vi "NIMS_NS_fir_nyquist.vi"(5 "Function name":string, 6 "Line number":i32, 7 "Number of outputs requested":i32, 8 "error in (no error)":errorcluster, 11 "[A]":variant[](array[variant])) -> (0 "error out":errorcluster, 3 "[funct(A)]":variant[](array[variant]))   [LabVIEW 2017]
uses:
  <vilib>/imath/engines/lvmath/Functions/Error Handling/error.ctl
  <instcachedir>/0/NIMS_RunTimeType_From StrictType (excl LVString)_1019F277F0A747EDBCA0F6C52CA54500.lvgen/NIMS_RunTimeType_From StrictType (excl LVString)_1019F277F0A747EDBCA0F6C52CA54500_000.vi
  <instcachedir>/0/NIMS_Get Row Vector_w Error - Matrix_7ECCFA0649AF47C08F6F0C496599EB01.lvgen/NIMS_Get Row Vector_w Error - Matrix_7ECCFA0649AF47C08F6F0C496599EB01_000.vi
  <instcachedir>/0/NIMS_Get Scalar_w Error_1987D997E87247DDAC16EA23A5E9E4FC.lvgen/NIMS_Get Scalar_w Error_1987D997E87247DDAC16EA23A5E9E4FC_000.vi
  <instcachedir>/0/NIMS_Get Scalar_w Error_1987D997E87247DDAC16EA23A5E9E4FC.lvgen/NIMS_Get Scalar_w Error_1987D997E87247DDAC16EA23A5E9E4FC_003.vi
  <instcachedir>/0/NIMS_Complex To Real_BE01396FDE034E8E94CEBBA1E368668D.lvgen/NIMS_Complex To Real_BE01396FDE034E8E94CEBBA1E368668D_000.vi
  <instcachedir>/0/NIMS_Get Row Vector_w Error - Matrix_7ECCFA0649AF47C08F6F0C496599EB01.lvgen/NIMS_Get Row Vector_w Error - Matrix_7ECCFA0649AF47C08F6F0C496599EB01_001.vi
  <instcachedir>/0/NIMS_RunTimeType_To Numeric_1CBDAFC4EFAD4045A1DE52278D16738D.lvgen/NIMS_RunTimeType_To Numeric_1CBDAFC4EFAD4045A1DE52278D16738D_000.vi
  <vilib>/addons/Digital Filter Design/NI_DigFilter_MathScript.lvlib
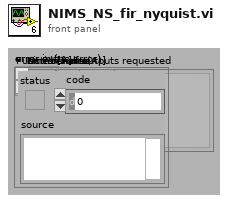
[diagram p1: front panel]
types:
  T1 = typedef "error.ctl" = enum16{"No Error", "Problem", "Input type must not be void", "Incorrect number of parameters", "Function not defined for non-numeric types", "An output variable of the user-defined function is undefined", "Function only defined for character arrays", "Function not defined for boolean, character, or single precision", "Function not defined for complex types", "Not a valid operation", "Inputs must be scalar", "Input matrices are not the same size", "Function only available on RT", "Input matrices must be nonnegative integers of the same type", "Arguments must be non-negative integers less than bitmax", "Number to complement must be less than 2^N", "Bit to get is outside range", "Bit to set is outside range", "Input must be real type ", "At least one parameter must be scalar", "Unable to display plug-in data on RT", "Function not defined for higher dimensional matrices", "Invalid attributes", "Wrong Type of Input Arguments", "Wrong Argument Option", "Invalid file identifier", "Indices must be real positive integers", "The variable is not a matrix data type.", "Number of elements must be the same for indices and values", "You cannot replace elements of a matrix with non-matrix data types.", "Cannot resize a 2D matrix with a linear index", "Unknown variable or symbol", "Indices out of range", "Empty matrix deletion can not be used with two indices", "Number of rows and columns must be the same for indices and values.", "Complex cannot be converted to Boolean", "Char cannot be converted to Boolean", "int64 cannot be converted to Boolean", "uint64 cannot be converted to Boolean", "You cannot convert a Boolean to a character.", "Incompatible input size in 3D surface function", "All rows must have the same number of columns", "Incompatible types", "Invalid matrix dimensions", "Dimension must be 1 or 2", "Base must be an integer between 2 and 36", "Invalid input", "Square matrix required", "Function 'timerstart' must be called before 'timerstop'", "Arguments must be positive real", "Step must not be zero", "Wrong number of input arguments", "Wrong number of output arguments", "Too many index arguments", "Input scalar must be >= 0", "Input scalar must be positive", "Input scalar must not be 0", "Input scalar must be in range [0,1]", "Can't use conditionally defined variable that's undefined", "Input must be a vector", "RT Exec Trace Toolkit not licensed", "Empty vector error", "All elements must be in domain [-1,1]", "All real elements of input vector must be >= 0", "All elements of input vector must be positive", "Values of input vectors are not compatible", "DAQmx not installed", "Input vector must be an increasing vector", "Dereferenced field does not exist within the struct", "A vector or matrix of structures must be indexed before it can be dereferenced", "Lenths of two input vectors are not compatible", "Invalid fieldname", "Empty matrix error", "Cannot use '.' on a type other than Struct", "Unused074", "Data type of the struct's field name is invalid", "Using . to dereference data that is not a struct", "Input struct contains invalid type ", "Size of input matrix is incompatible with input size", "Invalid format specifier", "Could not find field within struct", "Bad permutation array", "Mismatched fieldnames", "ode: User Function could not be opened", "ode: User Function signature does not meet ode requirements", "Unused085", "RunTime: MathScript could not be compiled", "Unknown function", "Only scalars and strings supported", "ode: User Function signature has incorrect number of inputs", "ode:User Function signature has incorrect number of outputs", "Range is too large", "End used without variable", "Function not available (RTE)", "Custom user error", "Arguments must be integers less than bitmax", "Shared library not found", "Header file not found", "Shared library already loaded", "Shared library not loaded", "Shared library function not found", "Shared library string return problem", "Problem calling shared library function", "Problem loading shared library from OS", "Problem parsing shared library header file", "Shared library incompatible types", "Shared library unsupported return type", "Shared library function not exported", "Shared library unsupported input type", "Problem unloading shared library from OS", "Function only available from UI", "Function specified in argument is missing", "An internal error has occurred", "Invalid object", "Invalid property", "Read-only property", "A break command has occurred", "A continue command has occurred", "A return command has occurred", "ode: times parameter invalid", "Function specified in argument has incorrect signature", "Function not found in file", "Reserved keyword cannot be defined as variable", "Reserved keyword cannot be defined as a function or script", "Arguments must be string literals", "Function not supported on this platform", "All columns must have the same number of rows", "Function ignored in RTE warning", "Cannot use : as a parameter that is not a variable", "Output can't be coerced to requested type", "Function not supported on current target", "Variable dependent on an unwired function input", "Unused132", "Unused133", "Unused134", "Unused135", "Unused136", "Unused137", "Unused138", "Unused139", "Global/Persistent must only take constants as arguments.", "Varargin must be last input in the function definition.", "Varargout must be last output in the function definition.", "Invalid output type. Cannot output a cell array of any type other than string.", "Invalid output type. Type is a dynamic struct.", "Invalid output type. Type is a struct that has a field whose type is not known until run-time", "Invalid output type. Type is a struct that has a field which is a plot object.", "MathScript parser DLL missing", "MathScript requires LabVIEW Full", "MathScript license is invalid or missing", "Varargout not supported except in assignments."}
  T2 = typedef "NIMS_CH_character datatype.ctl" = cluster{"Numeric":u8}
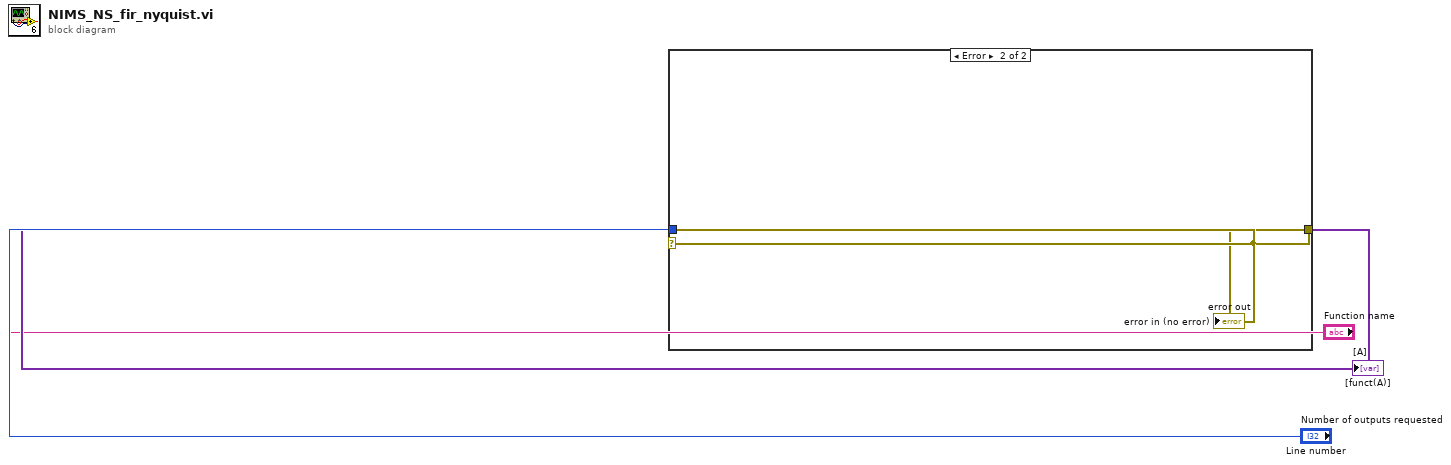
[diagram p0: block diagram]
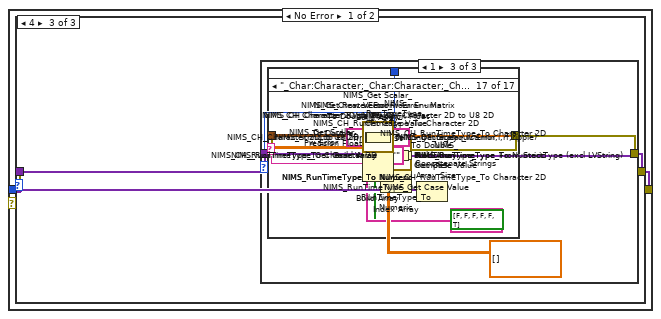
[diagram p2: hidden frame]
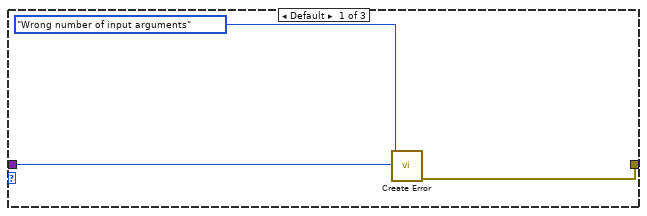
[diagram p3: hidden frame]
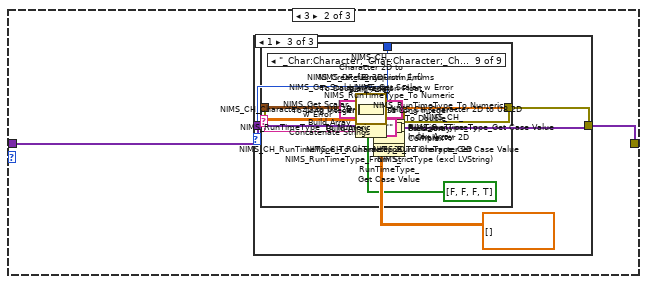
[diagram p4: hidden frame]
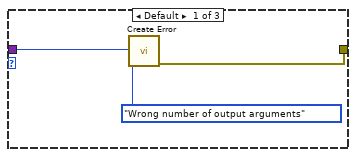
[diagram p5: hidden frame]
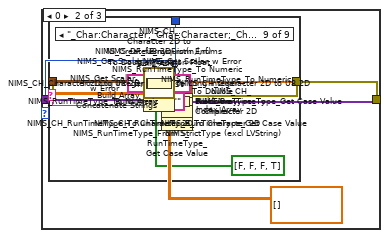
[diagram p6: hidden frame]
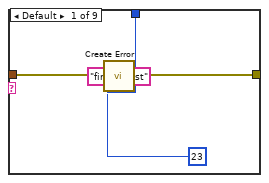
[diagram p7: hidden frame]
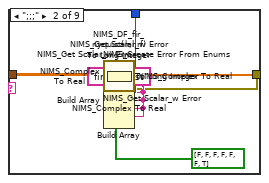
[diagram p8: hidden frame]
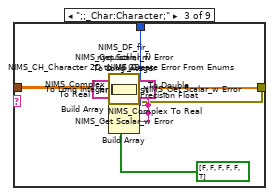
[diagram p9: hidden frame]
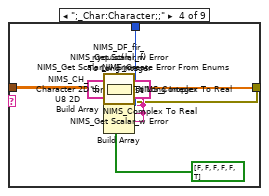
[diagram p10: hidden frame]
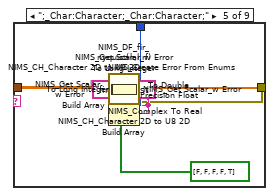
[diagram p11: hidden frame]
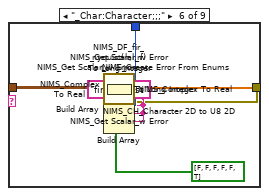
[diagram p12: hidden frame]
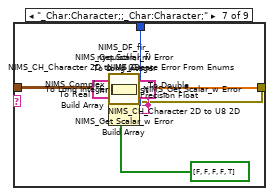
[diagram p13: hidden frame]
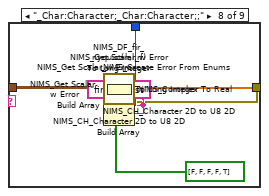
[diagram p14: hidden frame]
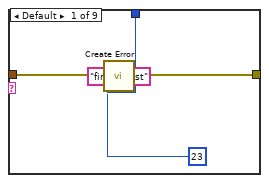
[diagram p15: hidden frame]
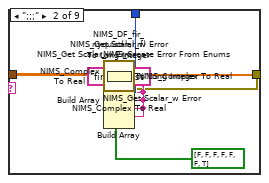
[diagram p16: hidden frame]
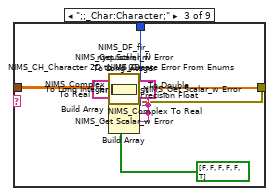
[diagram p17: hidden frame]
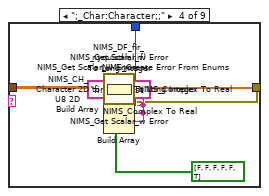
[diagram p18: hidden frame]
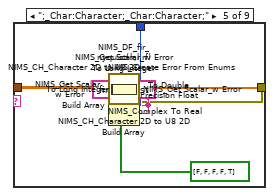
[diagram p19: hidden frame]
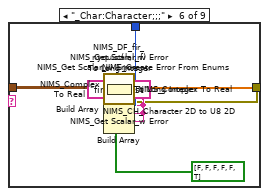
[diagram p20: hidden frame]
diagram:
  n1 = case shown="Error" "error in (no error)" {
    selector: "error in (no error)" -> [_ w1675]
    tunnel: [w15 _] -> w4
    tunnel: [w14 w1675] -> w3
    tunnel: "error in (no error)" -> [w13 _]
    tunnel: "Number of outputs requested" -> [w12 _]
    tunnel: "[A]" -> [w11 _]
    tunnel: "Function name" -> [w10 _]
    tunnel: "Line number" -> [w9 _]
    frame No Error {
      n2 = Array Size(array=w11) -> (size(s)=w8:i32)
      n3 = case shown="4" w8 {
        tunnel: [_ w27 w517] -> w15
        tunnel: w10 -> [w19 w24 w514]
        tunnel: w9 -> [w20 w25 w515]
        tunnel: w13 -> [w17 w23 w513]
        tunnel: [w16 w22 w512] -> w14
        tunnel: w12 -> [_ w21 w511]
        tunnel: w11 -> [_ w26 w516]
        frame Default {
          n4 = call <vilib>:"Create Error.vi"("Function name"=w19, "error in (no error)"=w17, "Error Enum"=error."Wrong number of input arguments", "Line number"=w20) -> ("error out"=w16:errorcluster)  [unwired: 6 in, 1 out]
        }
        frame 3 {
          n5 = case shown="1" w21 {
            tunnel: [_ w33 w272] -> w27
            tunnel: w24 -> [w31 _ _]
            tunnel: w25 -> [w32 w57 w296]
            tunnel: w23 -> [w29 w55 w294]
            tunnel: [w28 w39 w278] -> w22
            tunnel: w26 -> [_ w58 w297]
            frame Default {
              n6 = call <vilib>:"Create Error.vi"("Function name"=w31, "error in (no error)"=w29, "Error Enum"=error."Wrong number of output arguments", "Line number"=w32) -> ("error out"=w28:errorcluster)  [unwired: 6 in, 1 out]
            }
            frame 0 {
              n7 = Index Array(array=w58) -> (element #1=w54:variant, element #2=w49:variant, element #3=w44:variant)  [unwired: 3 in]
              n8 = call <vilib>:"NIMS_RunTimeType_Get Case Value.vi"("Data In"=w44) -> ("Case Value"=w40:string)  [unwired: 9 in, 1 out]
              n9 = call <vilib>:"NIMS_CH_RunTimeType_To Character 2D.vi"("Variant"=w44) -> ("data"=w41:T2[][])  [unwired: 1 in]
              n10 = call-generic <vilib>:"NIMS_RunTimeType_To Numeric.vi"("DataType"=cdb[][] [], "Variant"=w44) -> ("data"=w42:cdb[][])  [unwired: 1 in]
              n11 = call <vilib>:"NIMS_RunTimeType_Get Case Value.vi"("Data In"=w49) -> ("Case Value"=w45:string)  [unwired: 9 in, 1 out]
              n12 = call <vilib>:"NIMS_CH_RunTimeType_To Character 2D.vi"("Variant"=w49) -> ("data"=w46:T2[][])  [unwired: 1 in]
              n13 = call-generic <vilib>:"NIMS_RunTimeType_To Numeric.vi"("DataType"=cdb[][] [], "Variant"=w49) -> ("data"=w47:cdb[][])  [unwired: 1 in]
              n14 = call <vilib>:"NIMS_RunTimeType_Get Case Value.vi"("Data In"=w54) -> ("Case Value"=w50:string)  [unwired: 9 in, 1 out]
              n15 = call <vilib>:"NIMS_CH_RunTimeType_To Character 2D.vi"("Variant"=w54) -> ("data"=w51:T2[][])  [unwired: 1 in]
              n16 = call-generic <vilib>:"NIMS_RunTimeType_To Numeric.vi"("DataType"=cdb[][] [], "Variant"=w54) -> ("data"=w52:cdb[][])  [unwired: 1 in]
              n17 = Concatenate Strings(w50, w45, w40) -> (w56:string)
              n18 = case shown="\"_Char:Character;_Char:Character;_Char:Character;\"" w56 {
                tunnel: w55 -> [w60 w69 w96 w123 w149 w175 w201 w227 w252]
                tunnel: [_ w64 w91 w118 w144 w170 w196 w222 w247] -> w38
                tunnel: [w59 w65 w92 w119 w145 w171 w197 w223 w248] -> w39
                tunnel: w52 -> [_ w89 w116 w142 w168 _ _ _ _]
                tunnel: w51 -> [_ _ _ _ _ w194 w220 w245 w270]
                tunnel: w47 -> [_ w85 w112 _ _ w190 w216 _ _]
                tunnel: w46 -> [_ _ _ w138 w164 _ _ w241 w266]
                tunnel: w42 -> [_ w81 _ w134 _ w186 _ w237 _]
                tunnel: w41 -> [_ _ w108 _ w160 _ w212 _ w262]
                tunnel: w57 -> [w63 w72 w99 w126 w152 w178 w204 w230 w255]
                frame Default {
                  n19 = call <vilib>:"Create Error.vi"("Function name"="fir_nyquist", "error in (no error)"=w60, "Error Enum"=23, "Line number"=w63) -> ("error out"=w59:errorcluster)  [unwired: 6 in, 1 out]
                }
                frame ";;;" {
                  w67 = "fir_nyquist"
                  n20 = call-generic <vilib>:"NIMS_Complex To Real.vi"("A"=w81) -> ("Error Enum"=w75:T1, "Real(A)"=w80:dbl[][])  [unwired: 8 in, 1 out]
                  n21 = call-generic <vilib>:"NIMS_Get Scalar_w Error.vi"("A"=w80) -> ("Error Enum"=w74:T1, "Scalar"=w82:dbl)  [unwired: 8 in, 1 out]
                  n22 = call-generic <vilib>:"NIMS_Complex To Real.vi"("A"=w85) -> ("Error Enum"=w77:T1, "Real(A)"=w84:dbl[][])  [unwired: 8 in, 1 out]
                  n23 = To Long Integer(number=w84) -> (32bit integer=w83:i32[][])
                  n24 = call-generic <vilib>:"NIMS_Get Scalar_w Error.vi"("A"=w83) -> ("Error Enum"=w76:T1, "Scalar"=w86:i32)  [unwired: 8 in, 1 out]
                  n25 = call-generic <vilib>:"NIMS_Complex To Real.vi"("A"=w89) -> ("Error Enum"=w79:T1, "Real(A)"=w88:dbl[][])  [unwired: 8 in, 1 out]
                  n26 = To Long Integer(number=w88) -> (32bit integer=w87:i32[][])
                  n27 = call-generic <vilib>:"NIMS_Get Scalar_w Error.vi"("A"=w87) -> ("Error Enum"=w78:T1, "Scalar"=w90:i32)  [unwired: 8 in, 1 out]
                  n28 = call <vilib>:"NIMS_DF_fir_nyquist(n,l,rf).vi"("rolloff"=w82, "l"=w86, "n"=w90) -> ("error"=w73:i32, "b"=w64:dbl[])  [unwired: 7 in]
                  n29 = Build Array(w67, w67, w67, w67, w67, w67, "fir_nyquist") -> (w70:string[])
                  n30 = Build Array(w79, w78, w77, w76, w75, w74, w73) -> (w71:i32[])
                  n31 = call <vilib>:"NIMS_Create Error From Enums.vi"("Error Code"=bool[] [FALSE, FALSE, FALSE, FALSE, FALSE, FALSE, TRUE], "error in (no error)"=w69, "Line no"=w72, "Error Enums"=w71, "Function names"=w70) -> ("error out"=w65:errorcluster)  [unwired: 6 in]
                }
                frame ";;_Char:Character;" {
                  w94 = "fir_nyquist"
                  n32 = call <vilib>:"NIMS_CH_Character 2D to U8 2D.vi"("Character 2D array"=w108) -> ("U8 2D array"=w107:u8[][])  [unwired: 10 in]
                  n33 = To Double Precision Float(number=w107) -> (double precision float=w106:dbl[][])
                  n34 = call-generic <vilib>:"NIMS_Get Scalar_w Error.vi"("A"=w106) -> ("Error Enum"=w101:T1, "Scalar"=w109:dbl)  [unwired: 8 in, 1 out]
                  n35 = call-generic <vilib>:"NIMS_Complex To Real.vi"("A"=w112) -> ("Error Enum"=w103:T1, "Real(A)"=w111:dbl[][])  [unwired: 8 in, 1 out]
                  n36 = To Long Integer(number=w111) -> (32bit integer=w110:i32[][])
                  n37 = call-generic <vilib>:"NIMS_Get Scalar_w Error.vi"("A"=w110) -> ("Error Enum"=w102:T1, "Scalar"=w113:i32)  [unwired: 8 in, 1 out]
                  n38 = call-generic <vilib>:"NIMS_Complex To Real.vi"("A"=w116) -> ("Error Enum"=w105:T1, "Real(A)"=w115:dbl[][])  [unwired: 8 in, 1 out]
                  n39 = To Long Integer(number=w115) -> (32bit integer=w114:i32[][])
                  n40 = call-generic <vilib>:"NIMS_Get Scalar_w Error.vi"("A"=w114) -> ("Error Enum"=w104:T1, "Scalar"=w117:i32)  [unwired: 8 in, 1 out]
                  n41 = call <vilib>:"NIMS_DF_fir_nyquist(n,l,rf).vi"("rolloff"=w109, "l"=w113, "n"=w117) -> ("error"=w100:i32, "b"=w91:dbl[])  [unwired: 7 in]
                  n42 = Build Array(w94, w94, w94, w94, w94, "fir_nyquist") -> (w97:string[])
                  n43 = Build Array(w105, w104, w103, w102, w101, w100) -> (w98:i32[])
                  n44 = call <vilib>:"NIMS_Create Error From Enums.vi"("Error Code"=bool[] [FALSE, FALSE, FALSE, FALSE, FALSE, TRUE], "error in (no error)"=w96, "Line no"=w99, "Error Enums"=w98, "Function names"=w97) -> ("error out"=w92:errorcluster)  [unwired: 6 in]
                }
                frame ";_Char:Character;;" {
                  w121 = "fir_nyquist"
                  n45 = call-generic <vilib>:"NIMS_Complex To Real.vi"("A"=w134) -> ("Error Enum"=w129:T1, "Real(A)"=w133:dbl[][])  [unwired: 8 in, 1 out]
                  n46 = call-generic <vilib>:"NIMS_Get Scalar_w Error.vi"("A"=w133) -> ("Error Enum"=w128:T1, "Scalar"=w135:dbl)  [unwired: 8 in, 1 out]
                  n47 = call <vilib>:"NIMS_CH_Character 2D to U8 2D.vi"("Character 2D array"=w138) -> ("U8 2D array"=w137:u8[][])  [unwired: 10 in]
                  n48 = To Long Integer(number=w137) -> (32bit integer=w136:i32[][])
                  n49 = call-generic <vilib>:"NIMS_Get Scalar_w Error.vi"("A"=w136) -> ("Error Enum"=w130:T1, "Scalar"=w139:i32)  [unwired: 8 in, 1 out]
                  n50 = call-generic <vilib>:"NIMS_Complex To Real.vi"("A"=w142) -> ("Error Enum"=w132:T1, "Real(A)"=w141:dbl[][])  [unwired: 8 in, 1 out]
                  n51 = To Long Integer(number=w141) -> (32bit integer=w140:i32[][])
                  n52 = call-generic <vilib>:"NIMS_Get Scalar_w Error.vi"("A"=w140) -> ("Error Enum"=w131:T1, "Scalar"=w143:i32)  [unwired: 8 in, 1 out]
                  n53 = call <vilib>:"NIMS_DF_fir_nyquist(n,l,rf).vi"("rolloff"=w135, "l"=w139, "n"=w143) -> ("error"=w127:i32, "b"=w118:dbl[])  [unwired: 7 in]
                  n54 = Build Array(w121, w121, w121, w121, w121, "fir_nyquist") -> (w124:string[])
                  n55 = Build Array(w132, w131, w130, w129, w128, w127) -> (w125:i32[])
                  n56 = call <vilib>:"NIMS_Create Error From Enums.vi"("Error Code"=bool[] [FALSE, FALSE, FALSE, FALSE, FALSE, TRUE], "error in (no error)"=w123, "Line no"=w126, "Error Enums"=w125, "Function names"=w124) -> ("error out"=w119:errorcluster)  [unwired: 6 in]
                }
                frame ";_Char:Character;_Char:Character;" {
                  w147 = "fir_nyquist"
                  n57 = call <vilib>:"NIMS_CH_Character 2D to U8 2D.vi"("Character 2D array"=w160) -> ("U8 2D array"=w159:u8[][])  [unwired: 10 in]
                  n58 = To Double Precision Float(number=w159) -> (double precision float=w158:dbl[][])
                  n59 = call-generic <vilib>:"NIMS_Get Scalar_w Error.vi"("A"=w158) -> ("Error Enum"=w154:T1, "Scalar"=w161:dbl)  [unwired: 8 in, 1 out]
                  n60 = call <vilib>:"NIMS_CH_Character 2D to U8 2D.vi"("Character 2D array"=w164) -> ("U8 2D array"=w163:u8[][])  [unwired: 10 in]
                  n61 = To Long Integer(number=w163) -> (32bit integer=w162:i32[][])
                  n62 = call-generic <vilib>:"NIMS_Get Scalar_w Error.vi"("A"=w162) -> ("Error Enum"=w155:T1, "Scalar"=w165:i32)  [unwired: 8 in, 1 out]
                  n63 = call-generic <vilib>:"NIMS_Complex To Real.vi"("A"=w168) -> ("Error Enum"=w157:T1, "Real(A)"=w167:dbl[][])  [unwired: 8 in, 1 out]
                  n64 = To Long Integer(number=w167) -> (32bit integer=w166:i32[][])
                  n65 = call-generic <vilib>:"NIMS_Get Scalar_w Error.vi"("A"=w166) -> ("Error Enum"=w156:T1, "Scalar"=w169:i32)  [unwired: 8 in, 1 out]
                  n66 = call <vilib>:"NIMS_DF_fir_nyquist(n,l,rf).vi"("rolloff"=w161, "l"=w165, "n"=w169) -> ("error"=w153:i32, "b"=w144:dbl[])  [unwired: 7 in]
                  n67 = Build Array(w147, w147, w147, w147, "fir_nyquist") -> (w150:string[])
                  n68 = Build Array(w157, w156, w155, w154, w153) -> (w151:i32[])
                  n69 = call <vilib>:"NIMS_Create Error From Enums.vi"("Error Code"=bool[] [FALSE, FALSE, FALSE, FALSE, TRUE], "error in (no error)"=w149, "Line no"=w152, "Error Enums"=w151, "Function names"=w150) -> ("error out"=w145:errorcluster)  [unwired: 6 in]
                }
                frame "_Char:Character;;;" {
                  w173 = "fir_nyquist"
                  n70 = call-generic <vilib>:"NIMS_Complex To Real.vi"("A"=w186) -> ("Error Enum"=w181:T1, "Real(A)"=w185:dbl[][])  [unwired: 8 in, 1 out]
                  n71 = call-generic <vilib>:"NIMS_Get Scalar_w Error.vi"("A"=w185) -> ("Error Enum"=w180:T1, "Scalar"=w187:dbl)  [unwired: 8 in, 1 out]
                  n72 = call-generic <vilib>:"NIMS_Complex To Real.vi"("A"=w190) -> ("Error Enum"=w183:T1, "Real(A)"=w189:dbl[][])  [unwired: 8 in, 1 out]
                  n73 = To Long Integer(number=w189) -> (32bit integer=w188:i32[][])
                  n74 = call-generic <vilib>:"NIMS_Get Scalar_w Error.vi"("A"=w188) -> ("Error Enum"=w182:T1, "Scalar"=w191:i32)  [unwired: 8 in, 1 out]
                  n75 = call <vilib>:"NIMS_CH_Character 2D to U8 2D.vi"("Character 2D array"=w194) -> ("U8 2D array"=w193:u8[][])  [unwired: 10 in]
                  n76 = To Long Integer(number=w193) -> (32bit integer=w192:i32[][])
                  n77 = call-generic <vilib>:"NIMS_Get Scalar_w Error.vi"("A"=w192) -> ("Error Enum"=w184:T1, "Scalar"=w195:i32)  [unwired: 8 in, 1 out]
                  n78 = call <vilib>:"NIMS_DF_fir_nyquist(n,l,rf).vi"("rolloff"=w187, "l"=w191, "n"=w195) -> ("error"=w179:i32, "b"=w170:dbl[])  [unwired: 7 in]
                  n79 = Build Array(w173, w173, w173, w173, w173, "fir_nyquist") -> (w176:string[])
                  n80 = Build Array(w184, w183, w182, w181, w180, w179) -> (w177:i32[])
                  n81 = call <vilib>:"NIMS_Create Error From Enums.vi"("Error Code"=bool[] [FALSE, FALSE, FALSE, FALSE, FALSE, TRUE], "error in (no error)"=w175, "Line no"=w178, "Error Enums"=w177, "Function names"=w176) -> ("error out"=w171:errorcluster)  [unwired: 6 in]
                }
                frame "_Char:Character;;_Char:Character;" {
                  w199 = "fir_nyquist"
                  n82 = call <vilib>:"NIMS_CH_Character 2D to U8 2D.vi"("Character 2D array"=w212) -> ("U8 2D array"=w211:u8[][])  [unwired: 10 in]
                  n83 = To Double Precision Float(number=w211) -> (double precision float=w210:dbl[][])
                  n84 = call-generic <vilib>:"NIMS_Get Scalar_w Error.vi"("A"=w210) -> ("Error Enum"=w206:T1, "Scalar"=w213:dbl)  [unwired: 8 in, 1 out]
                  n85 = call-generic <vilib>:"NIMS_Complex To Real.vi"("A"=w216) -> ("Error Enum"=w208:T1, "Real(A)"=w215:dbl[][])  [unwired: 8 in, 1 out]
                  n86 = To Long Integer(number=w215) -> (32bit integer=w214:i32[][])
                  n87 = call-generic <vilib>:"NIMS_Get Scalar_w Error.vi"("A"=w214) -> ("Error Enum"=w207:T1, "Scalar"=w217:i32)  [unwired: 8 in, 1 out]
                  n88 = call <vilib>:"NIMS_CH_Character 2D to U8 2D.vi"("Character 2D array"=w220) -> ("U8 2D array"=w219:u8[][])  [unwired: 10 in]
                  n89 = To Long Integer(number=w219) -> (32bit integer=w218:i32[][])
                  n90 = call-generic <vilib>:"NIMS_Get Scalar_w Error.vi"("A"=w218) -> ("Error Enum"=w209:T1, "Scalar"=w221:i32)  [unwired: 8 in, 1 out]
                  n91 = call <vilib>:"NIMS_DF_fir_nyquist(n,l,rf).vi"("rolloff"=w213, "l"=w217, "n"=w221) -> ("error"=w205:i32, "b"=w196:dbl[])  [unwired: 7 in]
                  n92 = Build Array(w199, w199, w199, w199, "fir_nyquist") -> (w202:string[])
                  n93 = Build Array(w209, w208, w207, w206, w205) -> (w203:i32[])
                  n94 = call <vilib>:"NIMS_Create Error From Enums.vi"("Error Code"=bool[] [FALSE, FALSE, FALSE, FALSE, TRUE], "error in (no error)"=w201, "Line no"=w204, "Error Enums"=w203, "Function names"=w202) -> ("error out"=w197:errorcluster)  [unwired: 6 in]
                }
                frame "_Char:Character;_Char:Character;;" {
                  w225 = "fir_nyquist"
                  n95 = call-generic <vilib>:"NIMS_Complex To Real.vi"("A"=w237) -> ("Error Enum"=w233:T1, "Real(A)"=w236:dbl[][])  [unwired: 8 in, 1 out]
                  n96 = call-generic <vilib>:"NIMS_Get Scalar_w Error.vi"("A"=w236) -> ("Error Enum"=w232:T1, "Scalar"=w238:dbl)  [unwired: 8 in, 1 out]
                  n97 = call <vilib>:"NIMS_CH_Character 2D to U8 2D.vi"("Character 2D array"=w241) -> ("U8 2D array"=w240:u8[][])  [unwired: 10 in]
                  n98 = To Long Integer(number=w240) -> (32bit integer=w239:i32[][])
                  n99 = call-generic <vilib>:"NIMS_Get Scalar_w Error.vi"("A"=w239) -> ("Error Enum"=w234:T1, "Scalar"=w242:i32)  [unwired: 8 in, 1 out]
                  n100 = call <vilib>:"NIMS_CH_Character 2D to U8 2D.vi"("Character 2D array"=w245) -> ("U8 2D array"=w244:u8[][])  [unwired: 10 in]
                  n101 = To Long Integer(number=w244) -> (32bit integer=w243:i32[][])
                  n102 = call-generic <vilib>:"NIMS_Get Scalar_w Error.vi"("A"=w243) -> ("Error Enum"=w235:T1, "Scalar"=w246:i32)  [unwired: 8 in, 1 out]
                  n103 = call <vilib>:"NIMS_DF_fir_nyquist(n,l,rf).vi"("rolloff"=w238, "l"=w242, "n"=w246) -> ("error"=w231:i32, "b"=w222:dbl[])  [unwired: 7 in]
                  n104 = Build Array(w225, w225, w225, w225, "fir_nyquist") -> (w228:string[])
                  n105 = Build Array(w235, w234, w233, w232, w231) -> (w229:i32[])
                  n106 = call <vilib>:"NIMS_Create Error From Enums.vi"("Error Code"=bool[] [FALSE, FALSE, FALSE, FALSE, TRUE], "error in (no error)"=w227, "Line no"=w230, "Error Enums"=w229, "Function names"=w228) -> ("error out"=w223:errorcluster)  [unwired: 6 in]
                }
                frame "_Char:Character;_Char:Character;_Char:Character;" {
                  w250 = "fir_nyquist"
                  n107 = call <vilib>:"NIMS_CH_Character 2D to U8 2D.vi"("Character 2D array"=w262) -> ("U8 2D array"=w261:u8[][])  [unwired: 10 in]
                  n108 = To Double Precision Float(number=w261) -> (double precision float=w260:dbl[][])
                  n109 = call-generic <vilib>:"NIMS_Get Scalar_w Error.vi"("A"=w260) -> ("Error Enum"=w257:T1, "Scalar"=w263:dbl)  [unwired: 8 in, 1 out]
                  n110 = call <vilib>:"NIMS_CH_Character 2D to U8 2D.vi"("Character 2D array"=w266) -> ("U8 2D array"=w265:u8[][])  [unwired: 10 in]
                  n111 = To Long Integer(number=w265) -> (32bit integer=w264:i32[][])
                  n112 = call-generic <vilib>:"NIMS_Get Scalar_w Error.vi"("A"=w264) -> ("Error Enum"=w258:T1, "Scalar"=w267:i32)  [unwired: 8 in, 1 out]
                  n113 = call <vilib>:"NIMS_CH_Character 2D to U8 2D.vi"("Character 2D array"=w270) -> ("U8 2D array"=w269:u8[][])  [unwired: 10 in]
                  n114 = To Long Integer(number=w269) -> (32bit integer=w268:i32[][])
                  n115 = call-generic <vilib>:"NIMS_Get Scalar_w Error.vi"("A"=w268) -> ("Error Enum"=w259:T1, "Scalar"=w271:i32)  [unwired: 8 in, 1 out]
                  n116 = call <vilib>:"NIMS_DF_fir_nyquist(n,l,rf).vi"("rolloff"=w263, "l"=w267, "n"=w271) -> ("error"=w256:i32, "b"=w247:dbl[])  [unwired: 7 in]
                  n117 = Build Array(w250, w250, w250, "fir_nyquist") -> (w253:string[])
                  n118 = Build Array(w259, w258, w257, w256) -> (w254:i32[])
                  n119 = call <vilib>:"NIMS_Create Error From Enums.vi"("Error Code"=bool[] [FALSE, FALSE, FALSE, TRUE], "error in (no error)"=w252, "Line no"=w255, "Error Enums"=w254, "Function names"=w253) -> ("error out"=w248:errorcluster)  [unwired: 6 in]
                }
              }
              n120 = Build Array(w38) -> (w37:dbl[][])
              n121 = To Double Precision Complex(1:w37) -> (0:w36:cdb[][])
              n122 = call-generic <vilib>:"NIMS_RunTimeType_From StrictType (excl LVString).vi"("Plug-In Name"="", "Data In"=w36) -> ("Data Out"=w34:variant)  [unwired: 2 in]
              n123 = Build Array(w34) -> (w33:variant[])
            }
            frame 1 {
              n124 = Index Array(array=w297) -> (element #1=w293:variant, element #2=w288:variant, element #3=w283:variant)  [unwired: 3 in]
              n125 = call <vilib>:"NIMS_RunTimeType_Get Case Value.vi"("Data In"=w283) -> ("Case Value"=w279:string)  [unwired: 9 in, 1 out]
              n126 = call <vilib>:"NIMS_CH_RunTimeType_To Character 2D.vi"("Variant"=w283) -> ("data"=w280:T2[][])  [unwired: 1 in]
              n127 = call-generic <vilib>:"NIMS_RunTimeType_To Numeric.vi"("DataType"=cdb[][] [], "Variant"=w283) -> ("data"=w281:cdb[][])  [unwired: 1 in]
              n128 = call <vilib>:"NIMS_RunTimeType_Get Case Value.vi"("Data In"=w288) -> ("Case Value"=w284:string)  [unwired: 9 in, 1 out]
              n129 = call <vilib>:"NIMS_CH_RunTimeType_To Character 2D.vi"("Variant"=w288) -> ("data"=w285:T2[][])  [unwired: 1 in]
              n130 = call-generic <vilib>:"NIMS_RunTimeType_To Numeric.vi"("DataType"=cdb[][] [], "Variant"=w288) -> ("data"=w286:cdb[][])  [unwired: 1 in]
              n131 = call <vilib>:"NIMS_RunTimeType_Get Case Value.vi"("Data In"=w293) -> ("Case Value"=w289:string)  [unwired: 9 in, 1 out]
              n132 = call <vilib>:"NIMS_CH_RunTimeType_To Character 2D.vi"("Variant"=w293) -> ("data"=w290:T2[][])  [unwired: 1 in]
              n133 = call-generic <vilib>:"NIMS_RunTimeType_To Numeric.vi"("DataType"=cdb[][] [], "Variant"=w293) -> ("data"=w291:cdb[][])  [unwired: 1 in]
              n134 = Concatenate Strings(w289, w284, w279) -> (w295:string)
              n135 = case shown="\"_Char:Character;_Char:Character;_Char:Character;\"" w295 {
                tunnel: w294 -> [w299 w308 w335 w362 w388 w414 w440 w466 w491]
                tunnel: [_ w303 w330 w357 w383 w409 w435 w461 w486] -> w277
                tunnel: [w298 w304 w331 w358 w384 w410 w436 w462 w487] -> w278
                tunnel: w291 -> [_ w328 w355 w381 w407 _ _ _ _]
                tunnel: w290 -> [_ _ _ _ _ w433 w459 w484 w509]
                tunnel: w286 -> [_ w324 w351 _ _ w429 w455 _ _]
                tunnel: w285 -> [_ _ _ w377 w403 _ _ w480 w505]
                tunnel: w281 -> [_ w320 _ w373 _ w425 _ w476 _]
                tunnel: w280 -> [_ _ w347 _ w399 _ w451 _ w501]
                tunnel: w296 -> [w302 w311 w338 w365 w391 w417 w443 w469 w494]
                frame Default {
                  n136 = call <vilib>:"Create Error.vi"("Function name"="fir_nyquist", "error in (no error)"=w299, "Error Enum"=23, "Line number"=w302) -> ("error out"=w298:errorcluster)  [unwired: 6 in, 1 out]
                }
                frame ";;;" {
                  w306 = "fir_nyquist"
                  n137 = call-generic <vilib>:"NIMS_Complex To Real.vi"("A"=w320) -> ("Error Enum"=w314:T1, "Real(A)"=w319:dbl[][])  [unwired: 8 in, 1 out]
                  n138 = call-generic <vilib>:"NIMS_Get Scalar_w Error.vi"("A"=w319) -> ("Error Enum"=w313:T1, "Scalar"=w321:dbl)  [unwired: 8 in, 1 out]
                  n139 = call-generic <vilib>:"NIMS_Complex To Real.vi"("A"=w324) -> ("Error Enum"=w316:T1, "Real(A)"=w323:dbl[][])  [unwired: 8 in, 1 out]
                  n140 = To Long Integer(number=w323) -> (32bit integer=w322:i32[][])
                  n141 = call-generic <vilib>:"NIMS_Get Scalar_w Error.vi"("A"=w322) -> ("Error Enum"=w315:T1, "Scalar"=w325:i32)  [unwired: 8 in, 1 out]
                  n142 = call-generic <vilib>:"NIMS_Complex To Real.vi"("A"=w328) -> ("Error Enum"=w318:T1, "Real(A)"=w327:dbl[][])  [unwired: 8 in, 1 out]
                  n143 = To Long Integer(number=w327) -> (32bit integer=w326:i32[][])
                  n144 = call-generic <vilib>:"NIMS_Get Scalar_w Error.vi"("A"=w326) -> ("Error Enum"=w317:T1, "Scalar"=w329:i32)  [unwired: 8 in, 1 out]
                  n145 = call <vilib>:"NIMS_DF_fir_nyquist(n,l,rf).vi"("rolloff"=w321, "l"=w325, "n"=w329) -> ("error"=w312:i32, "b"=w303:dbl[])  [unwired: 7 in]
                  n146 = Build Array(w306, w306, w306, w306, w306, w306, "fir_nyquist") -> (w309:string[])
                  n147 = Build Array(w318, w317, w316, w315, w314, w313, w312) -> (w310:i32[])
                  n148 = call <vilib>:"NIMS_Create Error From Enums.vi"("Error Code"=bool[] [FALSE, FALSE, FALSE, FALSE, FALSE, FALSE, TRUE], "error in (no error)"=w308, "Line no"=w311, "Error Enums"=w310, "Function names"=w309) -> ("error out"=w304:errorcluster)  [unwired: 6 in]
                }
                frame ";;_Char:Character;" {
                  w333 = "fir_nyquist"
                  n149 = call <vilib>:"NIMS_CH_Character 2D to U8 2D.vi"("Character 2D array"=w347) -> ("U8 2D array"=w346:u8[][])  [unwired: 10 in]
                  n150 = To Double Precision Float(number=w346) -> (double precision float=w345:dbl[][])
                  n151 = call-generic <vilib>:"NIMS_Get Scalar_w Error.vi"("A"=w345) -> ("Error Enum"=w340:T1, "Scalar"=w348:dbl)  [unwired: 8 in, 1 out]
                  n152 = call-generic <vilib>:"NIMS_Complex To Real.vi"("A"=w351) -> ("Error Enum"=w342:T1, "Real(A)"=w350:dbl[][])  [unwired: 8 in, 1 out]
                  n153 = To Long Integer(number=w350) -> (32bit integer=w349:i32[][])
                  n154 = call-generic <vilib>:"NIMS_Get Scalar_w Error.vi"("A"=w349) -> ("Error Enum"=w341:T1, "Scalar"=w352:i32)  [unwired: 8 in, 1 out]
                  n155 = call-generic <vilib>:"NIMS_Complex To Real.vi"("A"=w355) -> ("Error Enum"=w344:T1, "Real(A)"=w354:dbl[][])  [unwired: 8 in, 1 out]
                  n156 = To Long Integer(number=w354) -> (32bit integer=w353:i32[][])
                  n157 = call-generic <vilib>:"NIMS_Get Scalar_w Error.vi"("A"=w353) -> ("Error Enum"=w343:T1, "Scalar"=w356:i32)  [unwired: 8 in, 1 out]
                  n158 = call <vilib>:"NIMS_DF_fir_nyquist(n,l,rf).vi"("rolloff"=w348, "l"=w352, "n"=w356) -> ("error"=w339:i32, "b"=w330:dbl[])  [unwired: 7 in]
                  n159 = Build Array(w333, w333, w333, w333, w333, "fir_nyquist") -> (w336:string[])
                  n160 = Build Array(w344, w343, w342, w341, w340, w339) -> (w337:i32[])
                  n161 = call <vilib>:"NIMS_Create Error From Enums.vi"("Error Code"=bool[] [FALSE, FALSE, FALSE, FALSE, FALSE, TRUE], "error in (no error)"=w335, "Line no"=w338, "Error Enums"=w337, "Function names"=w336) -> ("error out"=w331:errorcluster)  [unwired: 6 in]
                }
                frame ";_Char:Character;;" {
                  w360 = "fir_nyquist"
                  n162 = call-generic <vilib>:"NIMS_Complex To Real.vi"("A"=w373) -> ("Error Enum"=w368:T1, "Real(A)"=w372:dbl[][])  [unwired: 8 in, 1 out]
                  n163 = call-generic <vilib>:"NIMS_Get Scalar_w Error.vi"("A"=w372) -> ("Error Enum"=w367:T1, "Scalar"=w374:dbl)  [unwired: 8 in, 1 out]
                  n164 = call <vilib>:"NIMS_CH_Character 2D to U8 2D.vi"("Character 2D array"=w377) -> ("U8 2D array"=w376:u8[][])  [unwired: 10 in]
                  n165 = To Long Integer(number=w376) -> (32bit integer=w375:i32[][])
                  n166 = call-generic <vilib>:"NIMS_Get Scalar_w Error.vi"("A"=w375) -> ("Error Enum"=w369:T1, "Scalar"=w378:i32)  [unwired: 8 in, 1 out]
                  n167 = call-generic <vilib>:"NIMS_Complex To Real.vi"("A"=w381) -> ("Error Enum"=w371:T1, "Real(A)"=w380:dbl[][])  [unwired: 8 in, 1 out]
                  n168 = To Long Integer(number=w380) -> (32bit integer=w379:i32[][])
                  n169 = call-generic <vilib>:"NIMS_Get Scalar_w Error.vi"("A"=w379) -> ("Error Enum"=w370:T1, "Scalar"=w382:i32)  [unwired: 8 in, 1 out]
                  n170 = call <vilib>:"NIMS_DF_fir_nyquist(n,l,rf).vi"("rolloff"=w374, "l"=w378, "n"=w382) -> ("error"=w366:i32, "b"=w357:dbl[])  [unwired: 7 in]
                  n171 = Build Array(w360, w360, w360, w360, w360, "fir_nyquist") -> (w363:string[])
                  n172 = Build Array(w371, w370, w369, w368, w367, w366) -> (w364:i32[])
                  n173 = call <vilib>:"NIMS_Create Error From Enums.vi"("Error Code"=bool[] [FALSE, FALSE, FALSE, FALSE, FALSE, TRUE], "error in (no error)"=w362, "Line no"=w365, "Error Enums"=w364, "Function names"=w363) -> ("error out"=w358:errorcluster)  [unwired: 6 in]
                }
                frame ";_Char:Character;_Char:Character;" {
                  w386 = "fir_nyquist"
                  n174 = call <vilib>:"NIMS_CH_Character 2D to U8 2D.vi"("Character 2D array"=w399) -> ("U8 2D array"=w398:u8[][])  [unwired: 10 in]
                  n175 = To Double Precision Float(number=w398) -> (double precision float=w397:dbl[][])
                  n176 = call-generic <vilib>:"NIMS_Get Scalar_w Error.vi"("A"=w397) -> ("Error Enum"=w393:T1, "Scalar"=w400:dbl)  [unwired: 8 in, 1 out]
                  n177 = call <vilib>:"NIMS_CH_Character 2D to U8 2D.vi"("Character 2D array"=w403) -> ("U8 2D array"=w402:u8[][])  [unwired: 10 in]
                  n178 = To Long Integer(number=w402) -> (32bit integer=w401:i32[][])
                  n179 = call-generic <vilib>:"NIMS_Get Scalar_w Error.vi"("A"=w401) -> ("Error Enum"=w394:T1, "Scalar"=w404:i32)  [unwired: 8 in, 1 out]
                  n180 = call-generic <vilib>:"NIMS_Complex To Real.vi"("A"=w407) -> ("Error Enum"=w396:T1, "Real(A)"=w406:dbl[][])  [unwired: 8 in, 1 out]
                  n181 = To Long Integer(number=w406) -> (32bit integer=w405:i32[][])
                  n182 = call-generic <vilib>:"NIMS_Get Scalar_w Error.vi"("A"=w405) -> ("Error Enum"=w395:T1, "Scalar"=w408:i32)  [unwired: 8 in, 1 out]
                  n183 = call <vilib>:"NIMS_DF_fir_nyquist(n,l,rf).vi"("rolloff"=w400, "l"=w404, "n"=w408) -> ("error"=w392:i32, "b"=w383:dbl[])  [unwired: 7 in]
                  n184 = Build Array(w386, w386, w386, w386, "fir_nyquist") -> (w389:string[])
                  n185 = Build Array(w396, w395, w394, w393, w392) -> (w390:i32[])
                  n186 = call <vilib>:"NIMS_Create Error From Enums.vi"("Error Code"=bool[] [FALSE, FALSE, FALSE, FALSE, TRUE], "error in (no error)"=w388, "Line no"=w391, "Error Enums"=w390, "Function names"=w389) -> ("error out"=w384:errorcluster)  [unwired: 6 in]
                }
                frame "_Char:Character;;;" {
                  w412 = "fir_nyquist"
                  n187 = call-generic <vilib>:"NIMS_Complex To Real.vi"("A"=w425) -> ("Error Enum"=w420:T1, "Real(A)"=w424:dbl[][])  [unwired: 8 in, 1 out]
                  n188 = call-generic <vilib>:"NIMS_Get Scalar_w Error.vi"("A"=w424) -> ("Error Enum"=w419:T1, "Scalar"=w426:dbl)  [unwired: 8 in, 1 out]
                  n189 = call-generic <vilib>:"NIMS_Complex To Real.vi"("A"=w429) -> ("Error Enum"=w422:T1, "Real(A)"=w428:dbl[][])  [unwired: 8 in, 1 out]
                  n190 = To Long Integer(number=w428) -> (32bit integer=w427:i32[][])
                  n191 = call-generic <vilib>:"NIMS_Get Scalar_w Error.vi"("A"=w427) -> ("Error Enum"=w421:T1, "Scalar"=w430:i32)  [unwired: 8 in, 1 out]
                  n192 = call <vilib>:"NIMS_CH_Character 2D to U8 2D.vi"("Character 2D array"=w433) -> ("U8 2D array"=w432:u8[][])  [unwired: 10 in]
                  n193 = To Long Integer(number=w432) -> (32bit integer=w431:i32[][])
                  n194 = call-generic <vilib>:"NIMS_Get Scalar_w Error.vi"("A"=w431) -> ("Error Enum"=w423:T1, "Scalar"=w434:i32)  [unwired: 8 in, 1 out]
                  n195 = call <vilib>:"NIMS_DF_fir_nyquist(n,l,rf).vi"("rolloff"=w426, "l"=w430, "n"=w434) -> ("error"=w418:i32, "b"=w409:dbl[])  [unwired: 7 in]
                  n196 = Build Array(w412, w412, w412, w412, w412, "fir_nyquist") -> (w415:string[])
                  n197 = Build Array(w423, w422, w421, w420, w419, w418) -> (w416:i32[])
                  n198 = call <vilib>:"NIMS_Create Error From Enums.vi"("Error Code"=bool[] [FALSE, FALSE, FALSE, FALSE, FALSE, TRUE], "error in (no error)"=w414, "Line no"=w417, "Error Enums"=w416, "Function names"=w415) -> ("error out"=w410:errorcluster)  [unwired: 6 in]
                }
                frame "_Char:Character;;_Char:Character;" {
                  w438 = "fir_nyquist"
                  n199 = call <vilib>:"NIMS_CH_Character 2D to U8 2D.vi"("Character 2D array"=w451) -> ("U8 2D array"=w450:u8[][])  [unwired: 10 in]
                  n200 = To Double Precision Float(number=w450) -> (double precision float=w449:dbl[][])
                  n201 = call-generic <vilib>:"NIMS_Get Scalar_w Error.vi"("A"=w449) -> ("Error Enum"=w445:T1, "Scalar"=w452:dbl)  [unwired: 8 in, 1 out]
                  n202 = call-generic <vilib>:"NIMS_Complex To Real.vi"("A"=w455) -> ("Error Enum"=w447:T1, "Real(A)"=w454:dbl[][])  [unwired: 8 in, 1 out]
                  n203 = To Long Integer(number=w454) -> (32bit integer=w453:i32[][])
                  n204 = call-generic <vilib>:"NIMS_Get Scalar_w Error.vi"("A"=w453) -> ("Error Enum"=w446:T1, "Scalar"=w456:i32)  [unwired: 8 in, 1 out]
                  n205 = call <vilib>:"NIMS_CH_Character 2D to U8 2D.vi"("Character 2D array"=w459) -> ("U8 2D array"=w458:u8[][])  [unwired: 10 in]
                  n206 = To Long Integer(number=w458) -> (32bit integer=w457:i32[][])
                  n207 = call-generic <vilib>:"NIMS_Get Scalar_w Error.vi"("A"=w457) -> ("Error Enum"=w448:T1, "Scalar"=w460:i32)  [unwired: 8 in, 1 out]
                  n208 = call <vilib>:"NIMS_DF_fir_nyquist(n,l,rf).vi"("rolloff"=w452, "l"=w456, "n"=w460) -> ("error"=w444:i32, "b"=w435:dbl[])  [unwired: 7 in]
                  n209 = Build Array(w438, w438, w438, w438, "fir_nyquist") -> (w441:string[])
                  n210 = Build Array(w448, w447, w446, w445, w444) -> (w442:i32[])
                  n211 = call <vilib>:"NIMS_Create Error From Enums.vi"("Error Code"=bool[] [FALSE, FALSE, FALSE, FALSE, TRUE], "error in (no error)"=w440, "Line no"=w443, "Error Enums"=w442, "Function names"=w441) -> ("error out"=w436:errorcluster)  [unwired: 6 in]
                }
                frame "_Char:Character;_Char:Character;;" {
                  w464 = "fir_nyquist"
                  n212 = call-generic <vilib>:"NIMS_Complex To Real.vi"("A"=w476) -> ("Error Enum"=w472:T1, "Real(A)"=w475:dbl[][])  [unwired: 8 in, 1 out]
                  n213 = call-generic <vilib>:"NIMS_Get Scalar_w Error.vi"("A"=w475) -> ("Error Enum"=w471:T1, "Scalar"=w477:dbl)  [unwired: 8 in, 1 out]
                  n214 = call <vilib>:"NIMS_CH_Character 2D to U8 2D.vi"("Character 2D array"=w480) -> ("U8 2D array"=w479:u8[][])  [unwired: 10 in]
                  n215 = To Long Integer(number=w479) -> (32bit integer=w478:i32[][])
                  n216 = call-generic <vilib>:"NIMS_Get Scalar_w Error.vi"("A"=w478) -> ("Error Enum"=w473:T1, "Scalar"=w481:i32)  [unwired: 8 in, 1 out]
                  n217 = call <vilib>:"NIMS_CH_Character 2D to U8 2D.vi"("Character 2D array"=w484) -> ("U8 2D array"=w483:u8[][])  [unwired: 10 in]
                  n218 = To Long Integer(number=w483) -> (32bit integer=w482:i32[][])
                  n219 = call-generic <vilib>:"NIMS_Get Scalar_w Error.vi"("A"=w482) -> ("Error Enum"=w474:T1, "Scalar"=w485:i32)  [unwired: 8 in, 1 out]
                  n220 = call <vilib>:"NIMS_DF_fir_nyquist(n,l,rf).vi"("rolloff"=w477, "l"=w481, "n"=w485) -> ("error"=w470:i32, "b"=w461:dbl[])  [unwired: 7 in]
                  n221 = Build Array(w464, w464, w464, w464, "fir_nyquist") -> (w467:string[])
                  n222 = Build Array(w474, w473, w472, w471, w470) -> (w468:i32[])
                  n223 = call <vilib>:"NIMS_Create Error From Enums.vi"("Error Code"=bool[] [FALSE, FALSE, FALSE, FALSE, TRUE], "error in (no error)"=w466, "Line no"=w469, "Error Enums"=w468, "Function names"=w467) -> ("error out"=w462:errorcluster)  [unwired: 6 in]
                }
                frame "_Char:Character;_Char:Character;_Char:Character;" {
                  w489 = "fir_nyquist"
                  n224 = call <vilib>:"NIMS_CH_Character 2D to U8 2D.vi"("Character 2D array"=w501) -> ("U8 2D array"=w500:u8[][])  [unwired: 10 in]
                  n225 = To Double Precision Float(number=w500) -> (double precision float=w499:dbl[][])
                  n226 = call-generic <vilib>:"NIMS_Get Scalar_w Error.vi"("A"=w499) -> ("Error Enum"=w496:T1, "Scalar"=w502:dbl)  [unwired: 8 in, 1 out]
                  n227 = call <vilib>:"NIMS_CH_Character 2D to U8 2D.vi"("Character 2D array"=w505) -> ("U8 2D array"=w504:u8[][])  [unwired: 10 in]
                  n228 = To Long Integer(number=w504) -> (32bit integer=w503:i32[][])
                  n229 = call-generic <vilib>:"NIMS_Get Scalar_w Error.vi"("A"=w503) -> ("Error Enum"=w497:T1, "Scalar"=w506:i32)  [unwired: 8 in, 1 out]
                  n230 = call <vilib>:"NIMS_CH_Character 2D to U8 2D.vi"("Character 2D array"=w509) -> ("U8 2D array"=w508:u8[][])  [unwired: 10 in]
                  n231 = To Long Integer(number=w508) -> (32bit integer=w507:i32[][])
                  n232 = call-generic <vilib>:"NIMS_Get Scalar_w Error.vi"("A"=w507) -> ("Error Enum"=w498:T1, "Scalar"=w510:i32)  [unwired: 8 in, 1 out]
                  n233 = call <vilib>:"NIMS_DF_fir_nyquist(n,l,rf).vi"("rolloff"=w502, "l"=w506, "n"=w510) -> ("error"=w495:i32, "b"=w486:dbl[])  [unwired: 7 in]
                  n234 = Build Array(w489, w489, w489, "fir_nyquist") -> (w492:string[])
                  n235 = Build Array(w498, w497, w496, w495) -> (w493:i32[])
                  n236 = call <vilib>:"NIMS_Create Error From Enums.vi"("Error Code"=bool[] [FALSE, FALSE, FALSE, TRUE], "error in (no error)"=w491, "Line no"=w494, "Error Enums"=w493, "Function names"=w492) -> ("error out"=w487:errorcluster)  [unwired: 6 in]
                }
              }
              n237 = Build Array(w277) -> (w276:dbl[][])
              n238 = To Double Precision Complex(1:w276) -> (0:w275:cdb[][])
              n239 = call-generic <vilib>:"NIMS_RunTimeType_From StrictType (excl LVString).vi"("Plug-In Name"="", "Data In"=w275) -> ("Data Out"=w273:variant)  [unwired: 2 in]
              n240 = Build Array(w273) -> (w272:variant[])
            }
          }
        }
        frame 4 {
          n241 = case shown="1" w511 {
            tunnel: [_ w523 w1099] -> w517
            tunnel: w514 -> [w521 _ _]
            tunnel: w515 -> [w522 w552 w1128]
            tunnel: w513 -> [w519 w550 w1126]
            tunnel: [w518 w529 w1105] -> w512
            tunnel: w516 -> [_ w553 w1129]
            frame Default {
              n242 = call <vilib>:"Create Error.vi"("Function name"=w521, "error in (no error)"=w519, "Error Enum"=error."Wrong number of output arguments", "Line number"=w522) -> ("error out"=w518:errorcluster)  [unwired: 6 in, 1 out]
            }
            frame 0 {
              n243 = Index Array(array=w553) -> (element #1=w549:variant, element #2=w544:variant, element #3=w539:variant, element #4=w534:variant)  [unwired: 4 in]
              n244 = call <vilib>:"NIMS_RunTimeType_Get Case Value.vi"("Data In"=w534) -> ("Case Value"=w530:string)  [unwired: 9 in, 1 out]
              n245 = call <vilib>:"NIMS_CH_RunTimeType_To Character 2D.vi"("Variant"=w534) -> ("data"=w531:T2[][])  [unwired: 1 in]
              n246 = call-generic <vilib>:"NIMS_RunTimeType_To Numeric.vi"("DataType"=cdb[][] [], "Variant"=w534) -> ("data"=w532:cdb[][])  [unwired: 1 in]
              n247 = call <vilib>:"NIMS_RunTimeType_Get Case Value.vi"("Data In"=w539) -> ("Case Value"=w535:string)  [unwired: 9 in, 1 out]
              n248 = call <vilib>:"NIMS_CH_RunTimeType_To Character 2D.vi"("Variant"=w539) -> ("data"=w536:T2[][])  [unwired: 1 in]
              n249 = call-generic <vilib>:"NIMS_RunTimeType_To Numeric.vi"("DataType"=cdb[][] [], "Variant"=w539) -> ("data"=w537:cdb[][])  [unwired: 1 in]
              n250 = call <vilib>:"NIMS_RunTimeType_Get Case Value.vi"("Data In"=w544) -> ("Case Value"=w540:string)  [unwired: 9 in, 1 out]
              n251 = call <vilib>:"NIMS_CH_RunTimeType_To Character 2D.vi"("Variant"=w544) -> ("data"=w541:T2[][])  [unwired: 1 in]
              n252 = call-generic <vilib>:"NIMS_RunTimeType_To Numeric.vi"("DataType"=cdb[][] [], "Variant"=w544) -> ("data"=w542:cdb[][])  [unwired: 1 in]
              n253 = call <vilib>:"NIMS_RunTimeType_Get Case Value.vi"("Data In"=w549) -> ("Case Value"=w545:string)  [unwired: 9 in, 1 out]
              n254 = call <vilib>:"NIMS_CH_RunTimeType_To Character 2D.vi"("Variant"=w549) -> ("data"=w546:T2[][])  [unwired: 1 in]
              n255 = call-generic <vilib>:"NIMS_RunTimeType_To Numeric.vi"("DataType"=cdb[][] [], "Variant"=w549) -> ("data"=w547:cdb[][])  [unwired: 1 in]
              n256 = Concatenate Strings(w545, w540, w535, w530) -> (w551:string)
              n257 = case shown="\"_Char:Character;_Char:Character;_Char:Character;_Char:Character;\"" w551 {
                tunnel: w550 -> [w555 w564 w601 w635 w672 w706 w742 w775 w811 w844 w877 w910 w943 w976 w1008 w1040 w1072]
                tunnel: [_ w559 w596 w630 w667 w701 w737 w770 w806 w839 w872 w905 w938 w971 w1003 w1035 w1067] -> w528
                tunnel: [w554 w560 w597 w631 w668 w702 w738 w771 w807 w840 w873 w906 w939 w972 w1004 w1036 w1068] -> w529
                tunnel: w547 -> [_ w594 w628 w665 w699 w735 w768 w804 w837 _ _ _ _ _ _ _ _]
                tunnel: w546 -> [_ _ _ _ _ _ _ _ _ w869 w902 w935 w968 w1000 w1032 w1064 w1096]
                tunnel: w542 -> [_ w590 w624 w661 w695 _ _ _ _ w865 w898 w931 w964 _ _ _ _]
                tunnel: w541 -> [_ _ _ _ _ w731 w764 w800 w833 _ _ _ _ w996 w1028 w1060 w1092]
                tunnel: w537 -> [_ w586 w620 _ _ w727 w760 _ _ w861 w894 _ _ w992 w1024 _ _]
                tunnel: w536 -> [_ _ _ w657 w691 _ _ w796 w829 _ _ w927 w960 _ _ w1056 w1088]
                tunnel: w532 -> [_ w582 _ w652 _ w723 _ w791 _ w858 _ w923 _ w989 _ w1052 _]
                tunnel: w531 -> [_ _ w616 _ w686 _ w756 _ w824 _ w891 _ w956 _ w1021 _ w1084]
                tunnel: w552 -> [w558 w567 w604 w638 w675 w709 w745 w778 w814 w847 w880 w913 w946 w979 w1011 w1043 w1075]
                frame Default {
                  n258 = call <vilib>:"Create Error.vi"("Function name"="fir_nyquist", "error in (no error)"=w555, "Error Enum"=23, "Line number"=w558) -> ("error out"=w554:errorcluster)  [unwired: 6 in, 1 out]
                }
                frame ";;;;" {
                  w562 = "fir_nyquist"
                  n259 = call-generic <vilib>:"NIMS_Complex To Real.vi"("A"=w582) -> ("Error Enum"=w571:T1, "Real(A)"=w581:dbl[][])  [unwired: 8 in, 1 out]
                  n260 = To Unsigned Byte Integer(number=w581) -> (unsigned 8bit integer=w580:u8[][])
                  n261 = call-generic <vilib>:"NIMS_Get Row Vector_w Error - Matrix.vi"("A"=w580) -> ("Error Enum"=w570:T1, "Row Vector"=w579:u8[])  [unwired: 8 in, 1 out]
                  n262 = Byte Array To String(unsigned byte array=w579) -> (string=w583:string)
                  n263 = call <vilib>:"NIMS_String to Enum.vi"("Input String"=w583, "Enum choices"=string[] ["nonnegative"] ("Enum Options")) -> ("Error Enum"=w569:T1, "Enum Index"=w584:i32)  [unwired: 8 in]
                  n264 = call-generic <vilib>:"NIMS_Complex To Real.vi"("A"=w586) -> ("Error Enum"=w573:T1, "Real(A)"=w585:dbl[][])  [unwired: 8 in, 1 out]
                  n265 = call-generic <vilib>:"NIMS_Get Scalar_w Error.vi"("A"=w585) -> ("Error Enum"=w572:T1, "Scalar"=w587:dbl)  [unwired: 8 in, 1 out]
                  n266 = call-generic <vilib>:"NIMS_Complex To Real.vi"("A"=w590) -> ("Error Enum"=w575:T1, "Real(A)"=w589:dbl[][])  [unwired: 8 in, 1 out]
                  n267 = To Long Integer(number=w589) -> (32bit integer=w588:i32[][])
                  n268 = call-generic <vilib>:"NIMS_Get Scalar_w Error.vi"("A"=w588) -> ("Error Enum"=w574:T1, "Scalar"=w591:i32)  [unwired: 8 in, 1 out]
                  n269 = call-generic <vilib>:"NIMS_Complex To Real.vi"("A"=w594) -> ("Error Enum"=w577:T1, "Real(A)"=w593:dbl[][])  [unwired: 8 in, 1 out]
                  n270 = To Long Integer(number=w593) -> (32bit integer=w592:i32[][])
                  n271 = call-generic <vilib>:"NIMS_Get Scalar_w Error.vi"("A"=w592) -> ("Error Enum"=w576:T1, "Scalar"=w595:i32)  [unwired: 8 in, 1 out]
                  n272 = call <vilib>:"NIMS_DF_fir_nyquist(n,l,rf,non).vi"("flag"=w584, "rolloff"=w587, "l"=w591, "n"=w595) -> ("error"=w568:i32, "b"=w559:dbl[])  [unwired: 6 in]
                  n273 = Build Array(w562, w562, w562, w562, w562, w562, w562, w562, w562, "fir_nyquist") -> (w565:string[])
                  n274 = Build Array(w577, w576, w575, w574, w573, w572, w571, w570, w569, w568) -> (w566:i32[])
                  n275 = call <vilib>:"NIMS_Create Error From Enums.vi"("Error Code"=bool[] [FALSE, FALSE, FALSE, FALSE, FALSE, FALSE, FALSE, FALSE, FALSE, TRUE], "error in (no error)"=w564, "Line no"=w567, "Error Enums"=w566, "Function names"=w565) -> ("error out"=w560:errorcluster)  [unwired: 6 in]
                }
                frame ";;;_Char:Character;" {
                  w599 = "fir_nyquist"
                  n276 = call-generic <vilib>:"NIMS_Get Row Vector_w Error - Matrix.vi"("A"=w616) -> ("Error Enum"=w607:T1, "Row Vector"=w615:T2[])  [unwired: 8 in, 1 out]
                  n277 = call <vilib>:"NIMS_CH_Character RV to String.vi"("Character array"=w615) -> ("String"=w617:string)  [unwired: 10 in]
                  n278 = call <vilib>:"NIMS_String to Enum.vi"("Input String"=w617, "Enum choices"=string[] ["nonnegative"] ("Enum Options")) -> ("Error Enum"=w606:T1, "Enum Index"=w618:i32)  [unwired: 8 in]
                  n279 = call-generic <vilib>:"NIMS_Complex To Real.vi"("A"=w620) -> ("Error Enum"=w609:T1, "Real(A)"=w619:dbl[][])  [unwired: 8 in, 1 out]
                  n280 = call-generic <vilib>:"NIMS_Get Scalar_w Error.vi"("A"=w619) -> ("Error Enum"=w608:T1, "Scalar"=w621:dbl)  [unwired: 8 in, 1 out]
                  n281 = call-generic <vilib>:"NIMS_Complex To Real.vi"("A"=w624) -> ("Error Enum"=w611:T1, "Real(A)"=w623:dbl[][])  [unwired: 8 in, 1 out]
                  n282 = To Long Integer(number=w623) -> (32bit integer=w622:i32[][])
                  n283 = call-generic <vilib>:"NIMS_Get Scalar_w Error.vi"("A"=w622) -> ("Error Enum"=w610:T1, "Scalar"=w625:i32)  [unwired: 8 in, 1 out]
                  n284 = call-generic <vilib>:"NIMS_Complex To Real.vi"("A"=w628) -> ("Error Enum"=w613:T1, "Real(A)"=w627:dbl[][])  [unwired: 8 in, 1 out]
                  n285 = To Long Integer(number=w627) -> (32bit integer=w626:i32[][])
                  n286 = call-generic <vilib>:"NIMS_Get Scalar_w Error.vi"("A"=w626) -> ("Error Enum"=w612:T1, "Scalar"=w629:i32)  [unwired: 8 in, 1 out]
                  n287 = call <vilib>:"NIMS_DF_fir_nyquist(n,l,rf,non).vi"("flag"=w618, "rolloff"=w621, "l"=w625, "n"=w629) -> ("error"=w605:i32, "b"=w596:dbl[])  [unwired: 6 in]
                  n288 = Build Array(w599, w599, w599, w599, w599, w599, w599, w599, "fir_nyquist") -> (w602:string[])
                  n289 = Build Array(w613, w612, w611, w610, w609, w608, w607, w606, w605) -> (w603:i32[])
                  n290 = call <vilib>:"NIMS_Create Error From Enums.vi"("Error Code"=bool[] [FALSE, FALSE, FALSE, FALSE, FALSE, FALSE, FALSE, FALSE, TRUE], "error in (no error)"=w601, "Line no"=w604, "Error Enums"=w603, "Function names"=w602) -> ("error out"=w597:errorcluster)  [unwired: 6 in]
                }
                frame ";;_Char:Character;;" {
                  w633 = "fir_nyquist"
                  n291 = call-generic <vilib>:"NIMS_Complex To Real.vi"("A"=w652) -> ("Error Enum"=w642:T1, "Real(A)"=w651:dbl[][])  [unwired: 8 in, 1 out]
                  n292 = To Unsigned Byte Integer(number=w651) -> (unsigned 8bit integer=w650:u8[][])
                  n293 = call-generic <vilib>:"NIMS_Get Row Vector_w Error - Matrix.vi"("A"=w650) -> ("Error Enum"=w641:T1, "Row Vector"=w649:u8[])  [unwired: 8 in, 1 out]
                  n294 = Byte Array To String(unsigned byte array=w649) -> (string=w653:string)
                  n295 = call <vilib>:"NIMS_String to Enum.vi"("Input String"=w653, "Enum choices"=string[] ["nonnegative"] ("Enum Options")) -> ("Error Enum"=w640:T1, "Enum Index"=w654:i32)  [unwired: 8 in]
                  n296 = call <vilib>:"NIMS_CH_Character 2D to U8 2D.vi"("Character 2D array"=w657) -> ("U8 2D array"=w656:u8[][])  [unwired: 10 in]
                  n297 = To Double Precision Float(number=w656) -> (double precision float=w655:dbl[][])
                  n298 = call-generic <vilib>:"NIMS_Get Scalar_w Error.vi"("A"=w655) -> ("Error Enum"=w643:T1, "Scalar"=w658:dbl)  [unwired: 8 in, 1 out]
                  n299 = call-generic <vilib>:"NIMS_Complex To Real.vi"("A"=w661) -> ("Error Enum"=w645:T1, "Real(A)"=w660:dbl[][])  [unwired: 8 in, 1 out]
                  n300 = To Long Integer(number=w660) -> (32bit integer=w659:i32[][])
                  n301 = call-generic <vilib>:"NIMS_Get Scalar_w Error.vi"("A"=w659) -> ("Error Enum"=w644:T1, "Scalar"=w662:i32)  [unwired: 8 in, 1 out]
                  n302 = call-generic <vilib>:"NIMS_Complex To Real.vi"("A"=w665) -> ("Error Enum"=w647:T1, "Real(A)"=w664:dbl[][])  [unwired: 8 in, 1 out]
                  n303 = To Long Integer(number=w664) -> (32bit integer=w663:i32[][])
                  n304 = call-generic <vilib>:"NIMS_Get Scalar_w Error.vi"("A"=w663) -> ("Error Enum"=w646:T1, "Scalar"=w666:i32)  [unwired: 8 in, 1 out]
                  n305 = call <vilib>:"NIMS_DF_fir_nyquist(n,l,rf,non).vi"("flag"=w654, "rolloff"=w658, "l"=w662, "n"=w666) -> ("error"=w639:i32, "b"=w630:dbl[])  [unwired: 6 in]
                  n306 = Build Array(w633, w633, w633, w633, w633, w633, w633, w633, "fir_nyquist") -> (w636:string[])
                  n307 = Build Array(w647, w646, w645, w644, w643, w642, w641, w640, w639) -> (w637:i32[])
                  n308 = call <vilib>:"NIMS_Create Error From Enums.vi"("Error Code"=bool[] [FALSE, FALSE, FALSE, FALSE, FALSE, FALSE, FALSE, FALSE, TRUE], "error in (no error)"=w635, "Line no"=w638, "Error Enums"=w637, "Function names"=w636) -> ("error out"=w631:errorcluster)  [unwired: 6 in]
                }
                frame ";;_Char:Character;_Char:Character;" {
                  w670 = "fir_nyquist"
                  n309 = call-generic <vilib>:"NIMS_Get Row Vector_w Error - Matrix.vi"("A"=w686) -> ("Error Enum"=w678:T1, "Row Vector"=w685:T2[])  [unwired: 8 in, 1 out]
                  n310 = call <vilib>:"NIMS_CH_Character RV to String.vi"("Character array"=w685) -> ("String"=w687:string)  [unwired: 10 in]
                  n311 = call <vilib>:"NIMS_String to Enum.vi"("Input String"=w687, "Enum choices"=string[] ["nonnegative"] ("Enum Options")) -> ("Error Enum"=w677:T1, "Enum Index"=w688:i32)  [unwired: 8 in]
                  n312 = call <vilib>:"NIMS_CH_Character 2D to U8 2D.vi"("Character 2D array"=w691) -> ("U8 2D array"=w690:u8[][])  [unwired: 10 in]
                  n313 = To Double Precision Float(number=w690) -> (double precision float=w689:dbl[][])
                  n314 = call-generic <vilib>:"NIMS_Get Scalar_w Error.vi"("A"=w689) -> ("Error Enum"=w679:T1, "Scalar"=w692:dbl)  [unwired: 8 in, 1 out]
                  n315 = call-generic <vilib>:"NIMS_Complex To Real.vi"("A"=w695) -> ("Error Enum"=w681:T1, "Real(A)"=w694:dbl[][])  [unwired: 8 in, 1 out]
                  n316 = To Long Integer(number=w694) -> (32bit integer=w693:i32[][])
                  n317 = call-generic <vilib>:"NIMS_Get Scalar_w Error.vi"("A"=w693) -> ("Error Enum"=w680:T1, "Scalar"=w696:i32)  [unwired: 8 in, 1 out]
                  n318 = call-generic <vilib>:"NIMS_Complex To Real.vi"("A"=w699) -> ("Error Enum"=w683:T1, "Real(A)"=w698:dbl[][])  [unwired: 8 in, 1 out]
                  n319 = To Long Integer(number=w698) -> (32bit integer=w697:i32[][])
                  n320 = call-generic <vilib>:"NIMS_Get Scalar_w Error.vi"("A"=w697) -> ("Error Enum"=w682:T1, "Scalar"=w700:i32)  [unwired: 8 in, 1 out]
                  n321 = call <vilib>:"NIMS_DF_fir_nyquist(n,l,rf,non).vi"("flag"=w688, "rolloff"=w692, "l"=w696, "n"=w700) -> ("error"=w676:i32, "b"=w667:dbl[])  [unwired: 6 in]
                  n322 = Build Array(w670, w670, w670, w670, w670, w670, w670, "fir_nyquist") -> (w673:string[])
                  n323 = Build Array(w683, w682, w681, w680, w679, w678, w677, w676) -> (w674:i32[])
                  n324 = call <vilib>:"NIMS_Create Error From Enums.vi"("Error Code"=bool[] [FALSE, FALSE, FALSE, FALSE, FALSE, FALSE, FALSE, TRUE], "error in (no error)"=w672, "Line no"=w675, "Error Enums"=w674, "Function names"=w673) -> ("error out"=w668:errorcluster)  [unwired: 6 in]
                }
                frame ";_Char:Character;;;" {
                  w704 = "fir_nyquist"
                  n325 = call-generic <vilib>:"NIMS_Complex To Real.vi"("A"=w723) -> ("Error Enum"=w713:T1, "Real(A)"=w722:dbl[][])  [unwired: 8 in, 1 out]
                  n326 = To Unsigned Byte Integer(number=w722) -> (unsigned 8bit integer=w721:u8[][])
                  n327 = call-generic <vilib>:"NIMS_Get Row Vector_w Error - Matrix.vi"("A"=w721) -> ("Error Enum"=w712:T1, "Row Vector"=w720:u8[])  [unwired: 8 in, 1 out]
                  n328 = Byte Array To String(unsigned byte array=w720) -> (string=w724:string)
                  n329 = call <vilib>:"NIMS_String to Enum.vi"("Input String"=w724, "Enum choices"=string[] ["nonnegative"] ("Enum Options")) -> ("Error Enum"=w711:T1, "Enum Index"=w725:i32)  [unwired: 8 in]
                  n330 = call-generic <vilib>:"NIMS_Complex To Real.vi"("A"=w727) -> ("Error Enum"=w715:T1, "Real(A)"=w726:dbl[][])  [unwired: 8 in, 1 out]
                  n331 = call-generic <vilib>:"NIMS_Get Scalar_w Error.vi"("A"=w726) -> ("Error Enum"=w714:T1, "Scalar"=w728:dbl)  [unwired: 8 in, 1 out]
                  n332 = call <vilib>:"NIMS_CH_Character 2D to U8 2D.vi"("Character 2D array"=w731) -> ("U8 2D array"=w730:u8[][])  [unwired: 10 in]
                  n333 = To Long Integer(number=w730) -> (32bit integer=w729:i32[][])
                  n334 = call-generic <vilib>:"NIMS_Get Scalar_w Error.vi"("A"=w729) -> ("Error Enum"=w716:T1, "Scalar"=w732:i32)  [unwired: 8 in, 1 out]
                  n335 = call-generic <vilib>:"NIMS_Complex To Real.vi"("A"=w735) -> ("Error Enum"=w718:T1, "Real(A)"=w734:dbl[][])  [unwired: 8 in, 1 out]
                  n336 = To Long Integer(number=w734) -> (32bit integer=w733:i32[][])
                  n337 = call-generic <vilib>:"NIMS_Get Scalar_w Error.vi"("A"=w733) -> ("Error Enum"=w717:T1, "Scalar"=w736:i32)  [unwired: 8 in, 1 out]
                  n338 = call <vilib>:"NIMS_DF_fir_nyquist(n,l,rf,non).vi"("flag"=w725, "rolloff"=w728, "l"=w732, "n"=w736) -> ("error"=w710:i32, "b"=w701:dbl[])  [unwired: 6 in]
                  n339 = Build Array(w704, w704, w704, w704, w704, w704, w704, w704, "fir_nyquist") -> (w707:string[])
                  n340 = Build Array(w718, w717, w716, w715, w714, w713, w712, w711, w710) -> (w708:i32[])
                  n341 = call <vilib>:"NIMS_Create Error From Enums.vi"("Error Code"=bool[] [FALSE, FALSE, FALSE, FALSE, FALSE, FALSE, FALSE, FALSE, TRUE], "error in (no error)"=w706, "Line no"=w709, "Error Enums"=w708, "Function names"=w707) -> ("error out"=w702:errorcluster)  [unwired: 6 in]
                }
                frame ";_Char:Character;;_Char:Character;" {
                  w740 = "fir_nyquist"
                  n342 = call-generic <vilib>:"NIMS_Get Row Vector_w Error - Matrix.vi"("A"=w756) -> ("Error Enum"=w748:T1, "Row Vector"=w755:T2[])  [unwired: 8 in, 1 out]
                  n343 = call <vilib>:"NIMS_CH_Character RV to String.vi"("Character array"=w755) -> ("String"=w757:string)  [unwired: 10 in]
                  n344 = call <vilib>:"NIMS_String to Enum.vi"("Input String"=w757, "Enum choices"=string[] ["nonnegative"] ("Enum Options")) -> ("Error Enum"=w747:T1, "Enum Index"=w758:i32)  [unwired: 8 in]
                  n345 = call-generic <vilib>:"NIMS_Complex To Real.vi"("A"=w760) -> ("Error Enum"=w750:T1, "Real(A)"=w759:dbl[][])  [unwired: 8 in, 1 out]
                  n346 = call-generic <vilib>:"NIMS_Get Scalar_w Error.vi"("A"=w759) -> ("Error Enum"=w749:T1, "Scalar"=w761:dbl)  [unwired: 8 in, 1 out]
                  n347 = call <vilib>:"NIMS_CH_Character 2D to U8 2D.vi"("Character 2D array"=w764) -> ("U8 2D array"=w763:u8[][])  [unwired: 10 in]
                  n348 = To Long Integer(number=w763) -> (32bit integer=w762:i32[][])
                  n349 = call-generic <vilib>:"NIMS_Get Scalar_w Error.vi"("A"=w762) -> ("Error Enum"=w751:T1, "Scalar"=w765:i32)  [unwired: 8 in, 1 out]
                  n350 = call-generic <vilib>:"NIMS_Complex To Real.vi"("A"=w768) -> ("Error Enum"=w753:T1, "Real(A)"=w767:dbl[][])  [unwired: 8 in, 1 out]
                  n351 = To Long Integer(number=w767) -> (32bit integer=w766:i32[][])
                  n352 = call-generic <vilib>:"NIMS_Get Scalar_w Error.vi"("A"=w766) -> ("Error Enum"=w752:T1, "Scalar"=w769:i32)  [unwired: 8 in, 1 out]
                  n353 = call <vilib>:"NIMS_DF_fir_nyquist(n,l,rf,non).vi"("flag"=w758, "rolloff"=w761, "l"=w765, "n"=w769) -> ("error"=w746:i32, "b"=w737:dbl[])  [unwired: 6 in]
                  n354 = Build Array(w740, w740, w740, w740, w740, w740, w740, "fir_nyquist") -> (w743:string[])
                  n355 = Build Array(w753, w752, w751, w750, w749, w748, w747, w746) -> (w744:i32[])
                  n356 = call <vilib>:"NIMS_Create Error From Enums.vi"("Error Code"=bool[] [FALSE, FALSE, FALSE, FALSE, FALSE, FALSE, FALSE, TRUE], "error in (no error)"=w742, "Line no"=w745, "Error Enums"=w744, "Function names"=w743) -> ("error out"=w738:errorcluster)  [unwired: 6 in]
                }
                frame ";_Char:Character;_Char:Character;;" {
                  w773 = "fir_nyquist"
                  n357 = call-generic <vilib>:"NIMS_Complex To Real.vi"("A"=w791) -> ("Error Enum"=w782:T1, "Real(A)"=w790:dbl[][])  [unwired: 8 in, 1 out]
                  n358 = To Unsigned Byte Integer(number=w790) -> (unsigned 8bit integer=w789:u8[][])
                  n359 = call-generic <vilib>:"NIMS_Get Row Vector_w Error - Matrix.vi"("A"=w789) -> ("Error Enum"=w781:T1, "Row Vector"=w788:u8[])  [unwired: 8 in, 1 out]
                  n360 = Byte Array To String(unsigned byte array=w788) -> (string=w792:string)
                  n361 = call <vilib>:"NIMS_String to Enum.vi"("Input String"=w792, "Enum choices"=string[] ["nonnegative"] ("Enum Options")) -> ("Error Enum"=w780:T1, "Enum Index"=w793:i32)  [unwired: 8 in]
                  n362 = call <vilib>:"NIMS_CH_Character 2D to U8 2D.vi"("Character 2D array"=w796) -> ("U8 2D array"=w795:u8[][])  [unwired: 10 in]
                  n363 = To Double Precision Float(number=w795) -> (double precision float=w794:dbl[][])
                  n364 = call-generic <vilib>:"NIMS_Get Scalar_w Error.vi"("A"=w794) -> ("Error Enum"=w783:T1, "Scalar"=w797:dbl)  [unwired: 8 in, 1 out]
                  n365 = call <vilib>:"NIMS_CH_Character 2D to U8 2D.vi"("Character 2D array"=w800) -> ("U8 2D array"=w799:u8[][])  [unwired: 10 in]
                  n366 = To Long Integer(number=w799) -> (32bit integer=w798:i32[][])
                  n367 = call-generic <vilib>:"NIMS_Get Scalar_w Error.vi"("A"=w798) -> ("Error Enum"=w784:T1, "Scalar"=w801:i32)  [unwired: 8 in, 1 out]
                  n368 = call-generic <vilib>:"NIMS_Complex To Real.vi"("A"=w804) -> ("Error Enum"=w786:T1, "Real(A)"=w803:dbl[][])  [unwired: 8 in, 1 out]
                  n369 = To Long Integer(number=w803) -> (32bit integer=w802:i32[][])
                  n370 = call-generic <vilib>:"NIMS_Get Scalar_w Error.vi"("A"=w802) -> ("Error Enum"=w785:T1, "Scalar"=w805:i32)  [unwired: 8 in, 1 out]
                  n371 = call <vilib>:"NIMS_DF_fir_nyquist(n,l,rf,non).vi"("flag"=w793, "rolloff"=w797, "l"=w801, "n"=w805) -> ("error"=w779:i32, "b"=w770:dbl[])  [unwired: 6 in]
                  n372 = Build Array(w773, w773, w773, w773, w773, w773, w773, "fir_nyquist") -> (w776:string[])
                  n373 = Build Array(w786, w785, w784, w783, w782, w781, w780, w779) -> (w777:i32[])
                  n374 = call <vilib>:"NIMS_Create Error From Enums.vi"("Error Code"=bool[] [FALSE, FALSE, FALSE, FALSE, FALSE, FALSE, FALSE, TRUE], "error in (no error)"=w775, "Line no"=w778, "Error Enums"=w777, "Function names"=w776) -> ("error out"=w771:errorcluster)  [unwired: 6 in]
                }
                frame ";_Char:Character;_Char:Character;_Char:Character;" {
                  w809 = "fir_nyquist"
                  n375 = call-generic <vilib>:"NIMS_Get Row Vector_w Error - Matrix.vi"("A"=w824) -> ("Error Enum"=w817:T1, "Row Vector"=w823:T2[])  [unwired: 8 in, 1 out]
                  n376 = call <vilib>:"NIMS_CH_Character RV to String.vi"("Character array"=w823) -> ("String"=w825:string)  [unwired: 10 in]
                  n377 = call <vilib>:"NIMS_String to Enum.vi"("Input String"=w825, "Enum choices"=string[] ["nonnegative"] ("Enum Options")) -> ("Error Enum"=w816:T1, "Enum Index"=w826:i32)  [unwired: 8 in]
                  n378 = call <vilib>:"NIMS_CH_Character 2D to U8 2D.vi"("Character 2D array"=w829) -> ("U8 2D array"=w828:u8[][])  [unwired: 10 in]
                  n379 = To Double Precision Float(number=w828) -> (double precision float=w827:dbl[][])
                  n380 = call-generic <vilib>:"NIMS_Get Scalar_w Error.vi"("A"=w827) -> ("Error Enum"=w818:T1, "Scalar"=w830:dbl)  [unwired: 8 in, 1 out]
                  n381 = call <vilib>:"NIMS_CH_Character 2D to U8 2D.vi"("Character 2D array"=w833) -> ("U8 2D array"=w832:u8[][])  [unwired: 10 in]
                  n382 = To Long Integer(number=w832) -> (32bit integer=w831:i32[][])
                  n383 = call-generic <vilib>:"NIMS_Get Scalar_w Error.vi"("A"=w831) -> ("Error Enum"=w819:T1, "Scalar"=w834:i32)  [unwired: 8 in, 1 out]
                  n384 = call-generic <vilib>:"NIMS_Complex To Real.vi"("A"=w837) -> ("Error Enum"=w821:T1, "Real(A)"=w836:dbl[][])  [unwired: 8 in, 1 out]
                  n385 = To Long Integer(number=w836) -> (32bit integer=w835:i32[][])
                  n386 = call-generic <vilib>:"NIMS_Get Scalar_w Error.vi"("A"=w835) -> ("Error Enum"=w820:T1, "Scalar"=w838:i32)  [unwired: 8 in, 1 out]
                  n387 = call <vilib>:"NIMS_DF_fir_nyquist(n,l,rf,non).vi"("flag"=w826, "rolloff"=w830, "l"=w834, "n"=w838) -> ("error"=w815:i32, "b"=w806:dbl[])  [unwired: 6 in]
                  n388 = Build Array(w809, w809, w809, w809, w809, w809, "fir_nyquist") -> (w812:string[])
                  n389 = Build Array(w821, w820, w819, w818, w817, w816, w815) -> (w813:i32[])
                  n390 = call <vilib>:"NIMS_Create Error From Enums.vi"("Error Code"=bool[] [FALSE, FALSE, FALSE, FALSE, FALSE, FALSE, TRUE], "error in (no error)"=w811, "Line no"=w814, "Error Enums"=w813, "Function names"=w812) -> ("error out"=w807:errorcluster)  [unwired: 6 in]
                }
                frame "_Char:Character;;;;" {
                  w842 = "fir_nyquist"
                  n391 = call-generic <vilib>:"NIMS_Complex To Real.vi"("A"=w858) -> ("Error Enum"=w850:T1, "Real(A)"=w857:dbl[][])  [unwired: 8 in, 1 out]
                  n392 = call-generic <vilib>:"NIMS_Get Scalar_w Error.vi"("A"=w857) -> ("Error Enum"=w849:T1, "Scalar"=w859:dbl)  [unwired: 8 in, 1 out]
                  n393 = call-generic <vilib>:"NIMS_Complex To Real.vi"("A"=w861) -> ("Error Enum"=w852:T1, "Real(A)"=w860:dbl[][])  [unwired: 8 in, 1 out]
                  n394 = call-generic <vilib>:"NIMS_Get Scalar_w Error.vi"("A"=w860) -> ("Error Enum"=w851:T1, "Scalar"=w862:dbl)  [unwired: 8 in, 1 out]
                  n395 = call-generic <vilib>:"NIMS_Complex To Real.vi"("A"=w865) -> ("Error Enum"=w854:T1, "Real(A)"=w864:dbl[][])  [unwired: 8 in, 1 out]
                  n396 = To Long Integer(number=w864) -> (32bit integer=w863:i32[][])
                  n397 = call-generic <vilib>:"NIMS_Get Scalar_w Error.vi"("A"=w863) -> ("Error Enum"=w853:T1, "Scalar"=w866:i32)  [unwired: 8 in, 1 out]
                  n398 = call-generic <vilib>:"NIMS_Get Row Vector_w Error - Matrix.vi"("A"=w869) -> ("Error Enum"=w856:T1, "Row Vector"=w868:T2[])  [unwired: 8 in, 1 out]
                  n399 = call <vilib>:"NIMS_CH_Character RV to String.vi"("Character array"=w868) -> ("String"=w870:string)  [unwired: 10 in]
                  n400 = call <vilib>:"NIMS_String to Enum.vi"("Input String"=w870, "Enum choices"=string[] ["minorder"] ("Enum Options")) -> ("Error Enum"=w855:T1, "Enum Index"=w871:i32)  [unwired: 8 in]
                  n401 = call <vilib>:"NIMS_DF_fir_nyquist(min,l,rf,ripple).vi"("ripple"=w859, "rolloff"=w862, "l"=w866, "flag"=w871) -> ("error"=w848:i32, "b"=w839:dbl[])  [unwired: 6 in]
                  n402 = Build Array(w842, w842, w842, w842, w842, w842, w842, w842, "fir_nyquist") -> (w845:string[])
                  n403 = Build Array(w856, w855, w854, w853, w852, w851, w850, w849, w848) -> (w846:i32[])
                  n404 = call <vilib>:"NIMS_Create Error From Enums.vi"("Error Code"=bool[] [FALSE, FALSE, FALSE, FALSE, FALSE, FALSE, FALSE, FALSE, TRUE], "error in (no error)"=w844, "Line no"=w847, "Error Enums"=w846, "Function names"=w845) -> ("error out"=w840:errorcluster)  [unwired: 6 in]
                }
                frame "_Char:Character;;;_Char:Character;" {
                  w875 = "fir_nyquist"
                  n405 = call <vilib>:"NIMS_CH_Character 2D to U8 2D.vi"("Character 2D array"=w891) -> ("U8 2D array"=w890:u8[][])  [unwired: 10 in]
                  n406 = To Double Precision Float(number=w890) -> (double precision float=w889:dbl[][])
                  n407 = call-generic <vilib>:"NIMS_Get Scalar_w Error.vi"("A"=w889) -> ("Error Enum"=w882:T1, "Scalar"=w892:dbl)  [unwired: 8 in, 1 out]
                  n408 = call-generic <vilib>:"NIMS_Complex To Real.vi"("A"=w894) -> ("Error Enum"=w884:T1, "Real(A)"=w893:dbl[][])  [unwired: 8 in, 1 out]
                  n409 = call-generic <vilib>:"NIMS_Get Scalar_w Error.vi"("A"=w893) -> ("Error Enum"=w883:T1, "Scalar"=w895:dbl)  [unwired: 8 in, 1 out]
                  n410 = call-generic <vilib>:"NIMS_Complex To Real.vi"("A"=w898) -> ("Error Enum"=w886:T1, "Real(A)"=w897:dbl[][])  [unwired: 8 in, 1 out]
                  n411 = To Long Integer(number=w897) -> (32bit integer=w896:i32[][])
                  n412 = call-generic <vilib>:"NIMS_Get Scalar_w Error.vi"("A"=w896) -> ("Error Enum"=w885:T1, "Scalar"=w899:i32)  [unwired: 8 in, 1 out]
                  n413 = call-generic <vilib>:"NIMS_Get Row Vector_w Error - Matrix.vi"("A"=w902) -> ("Error Enum"=w888:T1, "Row Vector"=w901:T2[])  [unwired: 8 in, 1 out]
                  n414 = call <vilib>:"NIMS_CH_Character RV to String.vi"("Character array"=w901) -> ("String"=w903:string)  [unwired: 10 in]
                  n415 = call <vilib>:"NIMS_String to Enum.vi"("Input String"=w903, "Enum choices"=string[] ["minorder"] ("Enum Options")) -> ("Error Enum"=w887:T1, "Enum Index"=w904:i32)  [unwired: 8 in]
                  n416 = call <vilib>:"NIMS_DF_fir_nyquist(min,l,rf,ripple).vi"("ripple"=w892, "rolloff"=w895, "l"=w899, "flag"=w904) -> ("error"=w881:i32, "b"=w872:dbl[])  [unwired: 6 in]
                  n417 = Build Array(w875, w875, w875, w875, w875, w875, w875, "fir_nyquist") -> (w878:string[])
                  n418 = Build Array(w888, w887, w886, w885, w884, w883, w882, w881) -> (w879:i32[])
                  n419 = call <vilib>:"NIMS_Create Error From Enums.vi"("Error Code"=bool[] [FALSE, FALSE, FALSE, FALSE, FALSE, FALSE, FALSE, TRUE], "error in (no error)"=w877, "Line no"=w880, "Error Enums"=w879, "Function names"=w878) -> ("error out"=w873:errorcluster)  [unwired: 6 in]
                }
                frame "_Char:Character;;_Char:Character;;" {
                  w908 = "fir_nyquist"
                  n420 = call-generic <vilib>:"NIMS_Complex To Real.vi"("A"=w923) -> ("Error Enum"=w916:T1, "Real(A)"=w922:dbl[][])  [unwired: 8 in, 1 out]
                  n421 = call-generic <vilib>:"NIMS_Get Scalar_w Error.vi"("A"=w922) -> ("Error Enum"=w915:T1, "Scalar"=w924:dbl)  [unwired: 8 in, 1 out]
                  n422 = call <vilib>:"NIMS_CH_Character 2D to U8 2D.vi"("Character 2D array"=w927) -> ("U8 2D array"=w926:u8[][])  [unwired: 10 in]
                  n423 = To Double Precision Float(number=w926) -> (double precision float=w925:dbl[][])
                  n424 = call-generic <vilib>:"NIMS_Get Scalar_w Error.vi"("A"=w925) -> ("Error Enum"=w917:T1, "Scalar"=w928:dbl)  [unwired: 8 in, 1 out]
                  n425 = call-generic <vilib>:"NIMS_Complex To Real.vi"("A"=w931) -> ("Error Enum"=w919:T1, "Real(A)"=w930:dbl[][])  [unwired: 8 in, 1 out]
                  n426 = To Long Integer(number=w930) -> (32bit integer=w929:i32[][])
                  n427 = call-generic <vilib>:"NIMS_Get Scalar_w Error.vi"("A"=w929) -> ("Error Enum"=w918:T1, "Scalar"=w932:i32)  [unwired: 8 in, 1 out]
                  n428 = call-generic <vilib>:"NIMS_Get Row Vector_w Error - Matrix.vi"("A"=w935) -> ("Error Enum"=w921:T1, "Row Vector"=w934:T2[])  [unwired: 8 in, 1 out]
                  n429 = call <vilib>:"NIMS_CH_Character RV to String.vi"("Character array"=w934) -> ("String"=w936:string)  [unwired: 10 in]
                  n430 = call <vilib>:"NIMS_String to Enum.vi"("Input String"=w936, "Enum choices"=string[] ["minorder"] ("Enum Options")) -> ("Error Enum"=w920:T1, "Enum Index"=w937:i32)  [unwired: 8 in]
                  n431 = call <vilib>:"NIMS_DF_fir_nyquist(min,l,rf,ripple).vi"("ripple"=w924, "rolloff"=w928, "l"=w932, "flag"=w937) -> ("error"=w914:i32, "b"=w905:dbl[])  [unwired: 6 in]
                  n432 = Build Array(w908, w908, w908, w908, w908, w908, w908, "fir_nyquist") -> (w911:string[])
                  n433 = Build Array(w921, w920, w919, w918, w917, w916, w915, w914) -> (w912:i32[])
                  n434 = call <vilib>:"NIMS_Create Error From Enums.vi"("Error Code"=bool[] [FALSE, FALSE, FALSE, FALSE, FALSE, FALSE, FALSE, TRUE], "error in (no error)"=w910, "Line no"=w913, "Error Enums"=w912, "Function names"=w911) -> ("error out"=w906:errorcluster)  [unwired: 6 in]
                }
                frame "_Char:Character;;_Char:Character;_Char:Character;" {
                  w941 = "fir_nyquist"
                  n435 = call <vilib>:"NIMS_CH_Character 2D to U8 2D.vi"("Character 2D array"=w956) -> ("U8 2D array"=w955:u8[][])  [unwired: 10 in]
                  n436 = To Double Precision Float(number=w955) -> (double precision float=w954:dbl[][])
                  n437 = call-generic <vilib>:"NIMS_Get Scalar_w Error.vi"("A"=w954) -> ("Error Enum"=w948:T1, "Scalar"=w957:dbl)  [unwired: 8 in, 1 out]
                  n438 = call <vilib>:"NIMS_CH_Character 2D to U8 2D.vi"("Character 2D array"=w960) -> ("U8 2D array"=w959:u8[][])  [unwired: 10 in]
                  n439 = To Double Precision Float(number=w959) -> (double precision float=w958:dbl[][])
                  n440 = call-generic <vilib>:"NIMS_Get Scalar_w Error.vi"("A"=w958) -> ("Error Enum"=w949:T1, "Scalar"=w961:dbl)  [unwired: 8 in, 1 out]
                  n441 = call-generic <vilib>:"NIMS_Complex To Real.vi"("A"=w964) -> ("Error Enum"=w951:T1, "Real(A)"=w963:dbl[][])  [unwired: 8 in, 1 out]
                  n442 = To Long Integer(number=w963) -> (32bit integer=w962:i32[][])
                  n443 = call-generic <vilib>:"NIMS_Get Scalar_w Error.vi"("A"=w962) -> ("Error Enum"=w950:T1, "Scalar"=w965:i32)  [unwired: 8 in, 1 out]
                  n444 = call-generic <vilib>:"NIMS_Get Row Vector_w Error - Matrix.vi"("A"=w968) -> ("Error Enum"=w953:T1, "Row Vector"=w967:T2[])  [unwired: 8 in, 1 out]
                  n445 = call <vilib>:"NIMS_CH_Character RV to String.vi"("Character array"=w967) -> ("String"=w969:string)  [unwired: 10 in]
                  n446 = call <vilib>:"NIMS_String to Enum.vi"("Input String"=w969, "Enum choices"=string[] ["minorder"] ("Enum Options")) -> ("Error Enum"=w952:T1, "Enum Index"=w970:i32)  [unwired: 8 in]
                  n447 = call <vilib>:"NIMS_DF_fir_nyquist(min,l,rf,ripple).vi"("ripple"=w957, "rolloff"=w961, "l"=w965, "flag"=w970) -> ("error"=w947:i32, "b"=w938:dbl[])  [unwired: 6 in]
                  n448 = Build Array(w941, w941, w941, w941, w941, w941, "fir_nyquist") -> (w944:string[])
                  n449 = Build Array(w953, w952, w951, w950, w949, w948, w947) -> (w945:i32[])
                  n450 = call <vilib>:"NIMS_Create Error From Enums.vi"("Error Code"=bool[] [FALSE, FALSE, FALSE, FALSE, FALSE, FALSE, TRUE], "error in (no error)"=w943, "Line no"=w946, "Error Enums"=w945, "Function names"=w944) -> ("error out"=w939:errorcluster)  [unwired: 6 in]
                }
                frame "_Char:Character;_Char:Character;;;" {
                  w974 = "fir_nyquist"
                  n451 = call-generic <vilib>:"NIMS_Complex To Real.vi"("A"=w989) -> ("Error Enum"=w982:T1, "Real(A)"=w988:dbl[][])  [unwired: 8 in, 1 out]
                  n452 = call-generic <vilib>:"NIMS_Get Scalar_w Error.vi"("A"=w988) -> ("Error Enum"=w981:T1, "Scalar"=w990:dbl)  [unwired: 8 in, 1 out]
                  n453 = call-generic <vilib>:"NIMS_Complex To Real.vi"("A"=w992) -> ("Error Enum"=w984:T1, "Real(A)"=w991:dbl[][])  [unwired: 8 in, 1 out]
                  n454 = call-generic <vilib>:"NIMS_Get Scalar_w Error.vi"("A"=w991) -> ("Error Enum"=w983:T1, "Scalar"=w993:dbl)  [unwired: 8 in, 1 out]
                  n455 = call <vilib>:"NIMS_CH_Character 2D to U8 2D.vi"("Character 2D array"=w996) -> ("U8 2D array"=w995:u8[][])  [unwired: 10 in]
                  n456 = To Long Integer(number=w995) -> (32bit integer=w994:i32[][])
                  n457 = call-generic <vilib>:"NIMS_Get Scalar_w Error.vi"("A"=w994) -> ("Error Enum"=w985:T1, "Scalar"=w997:i32)  [unwired: 8 in, 1 out]
                  n458 = call-generic <vilib>:"NIMS_Get Row Vector_w Error - Matrix.vi"("A"=w1000) -> ("Error Enum"=w987:T1, "Row Vector"=w999:T2[])  [unwired: 8 in, 1 out]
                  n459 = call <vilib>:"NIMS_CH_Character RV to String.vi"("Character array"=w999) -> ("String"=w1001:string)  [unwired: 10 in]
                  n460 = call <vilib>:"NIMS_String to Enum.vi"("Input String"=w1001, "Enum choices"=string[] ["minorder"] ("Enum Options")) -> ("Error Enum"=w986:T1, "Enum Index"=w1002:i32)  [unwired: 8 in]
                  n461 = call <vilib>:"NIMS_DF_fir_nyquist(min,l,rf,ripple).vi"("ripple"=w990, "rolloff"=w993, "l"=w997, "flag"=w1002) -> ("error"=w980:i32, "b"=w971:dbl[])  [unwired: 6 in]
                  n462 = Build Array(w974, w974, w974, w974, w974, w974, w974, "fir_nyquist") -> (w977:string[])
                  n463 = Build Array(w987, w986, w985, w984, w983, w982, w981, w980) -> (w978:i32[])
                  n464 = call <vilib>:"NIMS_Create Error From Enums.vi"("Error Code"=bool[] [FALSE, FALSE, FALSE, FALSE, FALSE, FALSE, FALSE, TRUE], "error in (no error)"=w976, "Line no"=w979, "Error Enums"=w978, "Function names"=w977) -> ("error out"=w972:errorcluster)  [unwired: 6 in]
                }
                frame "_Char:Character;_Char:Character;;_Char:Character;" {
                  w1006 = "fir_nyquist"
                  n465 = call <vilib>:"NIMS_CH_Character 2D to U8 2D.vi"("Character 2D array"=w1021) -> ("U8 2D array"=w1020:u8[][])  [unwired: 10 in]
                  n466 = To Double Precision Float(number=w1020) -> (double precision float=w1019:dbl[][])
                  n467 = call-generic <vilib>:"NIMS_Get Scalar_w Error.vi"("A"=w1019) -> ("Error Enum"=w1013:T1, "Scalar"=w1022:dbl)  [unwired: 8 in, 1 out]
                  n468 = call-generic <vilib>:"NIMS_Complex To Real.vi"("A"=w1024) -> ("Error Enum"=w1015:T1, "Real(A)"=w1023:dbl[][])  [unwired: 8 in, 1 out]
                  n469 = call-generic <vilib>:"NIMS_Get Scalar_w Error.vi"("A"=w1023) -> ("Error Enum"=w1014:T1, "Scalar"=w1025:dbl)  [unwired: 8 in, 1 out]
                  n470 = call <vilib>:"NIMS_CH_Character 2D to U8 2D.vi"("Character 2D array"=w1028) -> ("U8 2D array"=w1027:u8[][])  [unwired: 10 in]
                  n471 = To Long Integer(number=w1027) -> (32bit integer=w1026:i32[][])
                  n472 = call-generic <vilib>:"NIMS_Get Scalar_w Error.vi"("A"=w1026) -> ("Error Enum"=w1016:T1, "Scalar"=w1029:i32)  [unwired: 8 in, 1 out]
                  n473 = call-generic <vilib>:"NIMS_Get Row Vector_w Error - Matrix.vi"("A"=w1032) -> ("Error Enum"=w1018:T1, "Row Vector"=w1031:T2[])  [unwired: 8 in, 1 out]
                  n474 = call <vilib>:"NIMS_CH_Character RV to String.vi"("Character array"=w1031) -> ("String"=w1033:string)  [unwired: 10 in]
                  n475 = call <vilib>:"NIMS_String to Enum.vi"("Input String"=w1033, "Enum choices"=string[] ["minorder"] ("Enum Options")) -> ("Error Enum"=w1017:T1, "Enum Index"=w1034:i32)  [unwired: 8 in]
                  n476 = call <vilib>:"NIMS_DF_fir_nyquist(min,l,rf,ripple).vi"("ripple"=w1022, "rolloff"=w1025, "l"=w1029, "flag"=w1034) -> ("error"=w1012:i32, "b"=w1003:dbl[])  [unwired: 6 in]
                  n477 = Build Array(w1006, w1006, w1006, w1006, w1006, w1006, "fir_nyquist") -> (w1009:string[])
                  n478 = Build Array(w1018, w1017, w1016, w1015, w1014, w1013, w1012) -> (w1010:i32[])
                  n479 = call <vilib>:"NIMS_Create Error From Enums.vi"("Error Code"=bool[] [FALSE, FALSE, FALSE, FALSE, FALSE, FALSE, TRUE], "error in (no error)"=w1008, "Line no"=w1011, "Error Enums"=w1010, "Function names"=w1009) -> ("error out"=w1004:errorcluster)  [unwired: 6 in]
                }
                frame "_Char:Character;_Char:Character;_Char:Character;;" {
                  w1038 = "fir_nyquist"
                  n480 = call-generic <vilib>:"NIMS_Complex To Real.vi"("A"=w1052) -> ("Error Enum"=w1046:T1, "Real(A)"=w1051:dbl[][])  [unwired: 8 in, 1 out]
                  n481 = call-generic <vilib>:"NIMS_Get Scalar_w Error.vi"("A"=w1051) -> ("Error Enum"=w1045:T1, "Scalar"=w1053:dbl)  [unwired: 8 in, 1 out]
                  n482 = call <vilib>:"NIMS_CH_Character 2D to U8 2D.vi"("Character 2D array"=w1056) -> ("U8 2D array"=w1055:u8[][])  [unwired: 10 in]
                  n483 = To Double Precision Float(number=w1055) -> (double precision float=w1054:dbl[][])
                  n484 = call-generic <vilib>:"NIMS_Get Scalar_w Error.vi"("A"=w1054) -> ("Error Enum"=w1047:T1, "Scalar"=w1057:dbl)  [unwired: 8 in, 1 out]
                  n485 = call <vilib>:"NIMS_CH_Character 2D to U8 2D.vi"("Character 2D array"=w1060) -> ("U8 2D array"=w1059:u8[][])  [unwired: 10 in]
                  n486 = To Long Integer(number=w1059) -> (32bit integer=w1058:i32[][])
                  n487 = call-generic <vilib>:"NIMS_Get Scalar_w Error.vi"("A"=w1058) -> ("Error Enum"=w1048:T1, "Scalar"=w1061:i32)  [unwired: 8 in, 1 out]
                  n488 = call-generic <vilib>:"NIMS_Get Row Vector_w Error - Matrix.vi"("A"=w1064) -> ("Error Enum"=w1050:T1, "Row Vector"=w1063:T2[])  [unwired: 8 in, 1 out]
                  n489 = call <vilib>:"NIMS_CH_Character RV to String.vi"("Character array"=w1063) -> ("String"=w1065:string)  [unwired: 10 in]
                  n490 = call <vilib>:"NIMS_String to Enum.vi"("Input String"=w1065, "Enum choices"=string[] ["minorder"] ("Enum Options")) -> ("Error Enum"=w1049:T1, "Enum Index"=w1066:i32)  [unwired: 8 in]
                  n491 = call <vilib>:"NIMS_DF_fir_nyquist(min,l,rf,ripple).vi"("ripple"=w1053, "rolloff"=w1057, "l"=w1061, "flag"=w1066) -> ("error"=w1044:i32, "b"=w1035:dbl[])  [unwired: 6 in]
                  n492 = Build Array(w1038, w1038, w1038, w1038, w1038, w1038, "fir_nyquist") -> (w1041:string[])
                  n493 = Build Array(w1050, w1049, w1048, w1047, w1046, w1045, w1044) -> (w1042:i32[])
                  n494 = call <vilib>:"NIMS_Create Error From Enums.vi"("Error Code"=bool[] [FALSE, FALSE, FALSE, FALSE, FALSE, FALSE, TRUE], "error in (no error)"=w1040, "Line no"=w1043, "Error Enums"=w1042, "Function names"=w1041) -> ("error out"=w1036:errorcluster)  [unwired: 6 in]
                }
                frame "_Char:Character;_Char:Character;_Char:Character;_Char:Character;" {
                  w1070 = "fir_nyquist"
                  n495 = call <vilib>:"NIMS_CH_Character 2D to U8 2D.vi"("Character 2D array"=w1084) -> ("U8 2D array"=w1083:u8[][])  [unwired: 10 in]
                  n496 = To Double Precision Float(number=w1083) -> (double precision float=w1082:dbl[][])
                  n497 = call-generic <vilib>:"NIMS_Get Scalar_w Error.vi"("A"=w1082) -> ("Error Enum"=w1077:T1, "Scalar"=w1085:dbl)  [unwired: 8 in, 1 out]
                  n498 = call <vilib>:"NIMS_CH_Character 2D to U8 2D.vi"("Character 2D array"=w1088) -> ("U8 2D array"=w1087:u8[][])  [unwired: 10 in]
                  n499 = To Double Precision Float(number=w1087) -> (double precision float=w1086:dbl[][])
                  n500 = call-generic <vilib>:"NIMS_Get Scalar_w Error.vi"("A"=w1086) -> ("Error Enum"=w1078:T1, "Scalar"=w1089:dbl)  [unwired: 8 in, 1 out]
                  n501 = call <vilib>:"NIMS_CH_Character 2D to U8 2D.vi"("Character 2D array"=w1092) -> ("U8 2D array"=w1091:u8[][])  [unwired: 10 in]
                  n502 = To Long Integer(number=w1091) -> (32bit integer=w1090:i32[][])
                  n503 = call-generic <vilib>:"NIMS_Get Scalar_w Error.vi"("A"=w1090) -> ("Error Enum"=w1079:T1, "Scalar"=w1093:i32)  [unwired: 8 in, 1 out]
                  n504 = call-generic <vilib>:"NIMS_Get Row Vector_w Error - Matrix.vi"("A"=w1096) -> ("Error Enum"=w1081:T1, "Row Vector"=w1095:T2[])  [unwired: 8 in, 1 out]
                  n505 = call <vilib>:"NIMS_CH_Character RV to String.vi"("Character array"=w1095) -> ("String"=w1097:string)  [unwired: 10 in]
                  n506 = call <vilib>:"NIMS_String to Enum.vi"("Input String"=w1097, "Enum choices"=string[] ["minorder"] ("Enum Options")) -> ("Error Enum"=w1080:T1, "Enum Index"=w1098:i32)  [unwired: 8 in]
                  n507 = call <vilib>:"NIMS_DF_fir_nyquist(min,l,rf,ripple).vi"("ripple"=w1085, "rolloff"=w1089, "l"=w1093, "flag"=w1098) -> ("error"=w1076:i32, "b"=w1067:dbl[])  [unwired: 6 in]
                  n508 = Build Array(w1070, w1070, w1070, w1070, w1070, "fir_nyquist") -> (w1073:string[])
                  n509 = Build Array(w1081, w1080, w1079, w1078, w1077, w1076) -> (w1074:i32[])
                  n510 = call <vilib>:"NIMS_Create Error From Enums.vi"("Error Code"=bool[] [FALSE, FALSE, FALSE, FALSE, FALSE, TRUE], "error in (no error)"=w1072, "Line no"=w1075, "Error Enums"=w1074, "Function names"=w1073) -> ("error out"=w1068:errorcluster)  [unwired: 6 in]
                }
              }
              n511 = Build Array(w528) -> (w527:dbl[][])
              n512 = To Double Precision Complex(1:w527) -> (0:w526:cdb[][])
              n513 = call-generic <vilib>:"NIMS_RunTimeType_From StrictType (excl LVString).vi"("Plug-In Name"="", "Data In"=w526) -> ("Data Out"=w524:variant)  [unwired: 2 in]
              n514 = Build Array(w524) -> (w523:variant[])
            }
            frame 1 {
              n515 = Index Array(array=w1129) -> (element #1=w1125:variant, element #2=w1120:variant, element #3=w1115:variant, element #4=w1110:variant)  [unwired: 4 in]
              n516 = call <vilib>:"NIMS_RunTimeType_Get Case Value.vi"("Data In"=w1110) -> ("Case Value"=w1106:string)  [unwired: 9 in, 1 out]
              n517 = call <vilib>:"NIMS_CH_RunTimeType_To Character 2D.vi"("Variant"=w1110) -> ("data"=w1107:T2[][])  [unwired: 1 in]
              n518 = call-generic <vilib>:"NIMS_RunTimeType_To Numeric.vi"("DataType"=cdb[][] [], "Variant"=w1110) -> ("data"=w1108:cdb[][])  [unwired: 1 in]
              n519 = call <vilib>:"NIMS_RunTimeType_Get Case Value.vi"("Data In"=w1115) -> ("Case Value"=w1111:string)  [unwired: 9 in, 1 out]
              n520 = call <vilib>:"NIMS_CH_RunTimeType_To Character 2D.vi"("Variant"=w1115) -> ("data"=w1112:T2[][])  [unwired: 1 in]
              n521 = call-generic <vilib>:"NIMS_RunTimeType_To Numeric.vi"("DataType"=cdb[][] [], "Variant"=w1115) -> ("data"=w1113:cdb[][])  [unwired: 1 in]
              n522 = call <vilib>:"NIMS_RunTimeType_Get Case Value.vi"("Data In"=w1120) -> ("Case Value"=w1116:string)  [unwired: 9 in, 1 out]
              n523 = call <vilib>:"NIMS_CH_RunTimeType_To Character 2D.vi"("Variant"=w1120) -> ("data"=w1117:T2[][])  [unwired: 1 in]
              n524 = call-generic <vilib>:"NIMS_RunTimeType_To Numeric.vi"("DataType"=cdb[][] [], "Variant"=w1120) -> ("data"=w1118:cdb[][])  [unwired: 1 in]
              n525 = call <vilib>:"NIMS_RunTimeType_Get Case Value.vi"("Data In"=w1125) -> ("Case Value"=w1121:string)  [unwired: 9 in, 1 out]
              n526 = call <vilib>:"NIMS_CH_RunTimeType_To Character 2D.vi"("Variant"=w1125) -> ("data"=w1122:T2[][])  [unwired: 1 in]
              n527 = call-generic <vilib>:"NIMS_RunTimeType_To Numeric.vi"("DataType"=cdb[][] [], "Variant"=w1125) -> ("data"=w1123:cdb[][])  [unwired: 1 in]
              n528 = Concatenate Strings(w1121, w1116, w1111, w1106) -> (w1127:string)
              n529 = case shown="\"_Char:Character;_Char:Character;_Char:Character;_Char:Character;\"" w1127 {
                tunnel: w1126 -> [w1131 w1140 w1177 w1211 w1248 w1282 w1318 w1351 w1387 w1420 w1453 w1486 w1519 w1552 w1584 w1616 w1648]
                tunnel: [_ w1135 w1172 w1206 w1243 w1277 w1313 w1346 w1382 w1415 w1448 w1481 w1514 w1547 w1579 w1611 w1643] -> w1104
                tunnel: [w1130 w1136 w1173 w1207 w1244 w1278 w1314 w1347 w1383 w1416 w1449 w1482 w1515 w1548 w1580 w1612 w1644] -> w1105
                tunnel: w1123 -> [_ w1170 w1204 w1241 w1275 w1311 w1344 w1380 w1413 _ _ _ _ _ _ _ _]
                tunnel: w1122 -> [_ _ _ _ _ _ _ _ _ w1445 w1478 w1511 w1544 w1576 w1608 w1640 w1672]
                tunnel: w1118 -> [_ w1166 w1200 w1237 w1271 _ _ _ _ w1441 w1474 w1507 w1540 _ _ _ _]
                tunnel: w1117 -> [_ _ _ _ _ w1307 w1340 w1376 w1409 _ _ _ _ w1572 w1604 w1636 w1668]
                tunnel: w1113 -> [_ w1162 w1196 _ _ w1303 w1336 _ _ w1437 w1470 _ _ w1568 w1600 _ _]
                tunnel: w1112 -> [_ _ _ w1233 w1267 _ _ w1372 w1405 _ _ w1503 w1536 _ _ w1632 w1664]
                tunnel: w1108 -> [_ w1158 _ w1228 _ w1299 _ w1367 _ w1434 _ w1499 _ w1565 _ w1628 _]
                tunnel: w1107 -> [_ _ w1192 _ w1262 _ w1332 _ w1400 _ w1467 _ w1532 _ w1597 _ w1660]
                tunnel: w1128 -> [w1134 w1143 w1180 w1214 w1251 w1285 w1321 w1354 w1390 w1423 w1456 w1489 w1522 w1555 w1587 w1619 w1651]
                frame Default {
                  n530 = call <vilib>:"Create Error.vi"("Function name"="fir_nyquist", "error in (no error)"=w1131, "Error Enum"=23, "Line number"=w1134) -> ("error out"=w1130:errorcluster)  [unwired: 6 in, 1 out]
                }
                frame ";;;;" {
                  w1138 = "fir_nyquist"
                  n531 = call-generic <vilib>:"NIMS_Complex To Real.vi"("A"=w1158) -> ("Error Enum"=w1147:T1, "Real(A)"=w1157:dbl[][])  [unwired: 8 in, 1 out]
                  n532 = To Unsigned Byte Integer(number=w1157) -> (unsigned 8bit integer=w1156:u8[][])
                  n533 = call-generic <vilib>:"NIMS_Get Row Vector_w Error - Matrix.vi"("A"=w1156) -> ("Error Enum"=w1146:T1, "Row Vector"=w1155:u8[])  [unwired: 8 in, 1 out]
                  n534 = Byte Array To String(unsigned byte array=w1155) -> (string=w1159:string)
                  n535 = call <vilib>:"NIMS_String to Enum.vi"("Input String"=w1159, "Enum choices"=string[] ["nonnegative"] ("Enum Options")) -> ("Error Enum"=w1145:T1, "Enum Index"=w1160:i32)  [unwired: 8 in]
                  n536 = call-generic <vilib>:"NIMS_Complex To Real.vi"("A"=w1162) -> ("Error Enum"=w1149:T1, "Real(A)"=w1161:dbl[][])  [unwired: 8 in, 1 out]
                  n537 = call-generic <vilib>:"NIMS_Get Scalar_w Error.vi"("A"=w1161) -> ("Error Enum"=w1148:T1, "Scalar"=w1163:dbl)  [unwired: 8 in, 1 out]
                  n538 = call-generic <vilib>:"NIMS_Complex To Real.vi"("A"=w1166) -> ("Error Enum"=w1151:T1, "Real(A)"=w1165:dbl[][])  [unwired: 8 in, 1 out]
                  n539 = To Long Integer(number=w1165) -> (32bit integer=w1164:i32[][])
                  n540 = call-generic <vilib>:"NIMS_Get Scalar_w Error.vi"("A"=w1164) -> ("Error Enum"=w1150:T1, "Scalar"=w1167:i32)  [unwired: 8 in, 1 out]
                  n541 = call-generic <vilib>:"NIMS_Complex To Real.vi"("A"=w1170) -> ("Error Enum"=w1153:T1, "Real(A)"=w1169:dbl[][])  [unwired: 8 in, 1 out]
                  n542 = To Long Integer(number=w1169) -> (32bit integer=w1168:i32[][])
                  n543 = call-generic <vilib>:"NIMS_Get Scalar_w Error.vi"("A"=w1168) -> ("Error Enum"=w1152:T1, "Scalar"=w1171:i32)  [unwired: 8 in, 1 out]
                  n544 = call <vilib>:"NIMS_DF_fir_nyquist(n,l,rf,non).vi"("flag"=w1160, "rolloff"=w1163, "l"=w1167, "n"=w1171) -> ("error"=w1144:i32, "b"=w1135:dbl[])  [unwired: 6 in]
                  n545 = Build Array(w1138, w1138, w1138, w1138, w1138, w1138, w1138, w1138, w1138, "fir_nyquist") -> (w1141:string[])
                  n546 = Build Array(w1153, w1152, w1151, w1150, w1149, w1148, w1147, w1146, w1145, w1144) -> (w1142:i32[])
                  n547 = call <vilib>:"NIMS_Create Error From Enums.vi"("Error Code"=bool[] [FALSE, FALSE, FALSE, FALSE, FALSE, FALSE, FALSE, FALSE, FALSE, TRUE], "error in (no error)"=w1140, "Line no"=w1143, "Error Enums"=w1142, "Function names"=w1141) -> ("error out"=w1136:errorcluster)  [unwired: 6 in]
                }
                frame ";;;_Char:Character;" {
                  w1175 = "fir_nyquist"
                  n548 = call-generic <vilib>:"NIMS_Get Row Vector_w Error - Matrix.vi"("A"=w1192) -> ("Error Enum"=w1183:T1, "Row Vector"=w1191:T2[])  [unwired: 8 in, 1 out]
                  n549 = call <vilib>:"NIMS_CH_Character RV to String.vi"("Character array"=w1191) -> ("String"=w1193:string)  [unwired: 10 in]
                  n550 = call <vilib>:"NIMS_String to Enum.vi"("Input String"=w1193, "Enum choices"=string[] ["nonnegative"] ("Enum Options")) -> ("Error Enum"=w1182:T1, "Enum Index"=w1194:i32)  [unwired: 8 in]
                  n551 = call-generic <vilib>:"NIMS_Complex To Real.vi"("A"=w1196) -> ("Error Enum"=w1185:T1, "Real(A)"=w1195:dbl[][])  [unwired: 8 in, 1 out]
                  n552 = call-generic <vilib>:"NIMS_Get Scalar_w Error.vi"("A"=w1195) -> ("Error Enum"=w1184:T1, "Scalar"=w1197:dbl)  [unwired: 8 in, 1 out]
                  n553 = call-generic <vilib>:"NIMS_Complex To Real.vi"("A"=w1200) -> ("Error Enum"=w1187:T1, "Real(A)"=w1199:dbl[][])  [unwired: 8 in, 1 out]
                  n554 = To Long Integer(number=w1199) -> (32bit integer=w1198:i32[][])
                  n555 = call-generic <vilib>:"NIMS_Get Scalar_w Error.vi"("A"=w1198) -> ("Error Enum"=w1186:T1, "Scalar"=w1201:i32)  [unwired: 8 in, 1 out]
                  n556 = call-generic <vilib>:"NIMS_Complex To Real.vi"("A"=w1204) -> ("Error Enum"=w1189:T1, "Real(A)"=w1203:dbl[][])  [unwired: 8 in, 1 out]
                  n557 = To Long Integer(number=w1203) -> (32bit integer=w1202:i32[][])
                  n558 = call-generic <vilib>:"NIMS_Get Scalar_w Error.vi"("A"=w1202) -> ("Error Enum"=w1188:T1, "Scalar"=w1205:i32)  [unwired: 8 in, 1 out]
                  n559 = call <vilib>:"NIMS_DF_fir_nyquist(n,l,rf,non).vi"("flag"=w1194, "rolloff"=w1197, "l"=w1201, "n"=w1205) -> ("error"=w1181:i32, "b"=w1172:dbl[])  [unwired: 6 in]
                  n560 = Build Array(w1175, w1175, w1175, w1175, w1175, w1175, w1175, w1175, "fir_nyquist") -> (w1178:string[])
                  n561 = Build Array(w1189, w1188, w1187, w1186, w1185, w1184, w1183, w1182, w1181) -> (w1179:i32[])
                  n562 = call <vilib>:"NIMS_Create Error From Enums.vi"("Error Code"=bool[] [FALSE, FALSE, FALSE, FALSE, FALSE, FALSE, FALSE, FALSE, TRUE], "error in (no error)"=w1177, "Line no"=w1180, "Error Enums"=w1179, "Function names"=w1178) -> ("error out"=w1173:errorcluster)  [unwired: 6 in]
                }
                frame ";;_Char:Character;;" {
                  w1209 = "fir_nyquist"
                  n563 = call-generic <vilib>:"NIMS_Complex To Real.vi"("A"=w1228) -> ("Error Enum"=w1218:T1, "Real(A)"=w1227:dbl[][])  [unwired: 8 in, 1 out]
                  n564 = To Unsigned Byte Integer(number=w1227) -> (unsigned 8bit integer=w1226:u8[][])
                  n565 = call-generic <vilib>:"NIMS_Get Row Vector_w Error - Matrix.vi"("A"=w1226) -> ("Error Enum"=w1217:T1, "Row Vector"=w1225:u8[])  [unwired: 8 in, 1 out]
                  n566 = Byte Array To String(unsigned byte array=w1225) -> (string=w1229:string)
                  n567 = call <vilib>:"NIMS_String to Enum.vi"("Input String"=w1229, "Enum choices"=string[] ["nonnegative"] ("Enum Options")) -> ("Error Enum"=w1216:T1, "Enum Index"=w1230:i32)  [unwired: 8 in]
                  n568 = call <vilib>:"NIMS_CH_Character 2D to U8 2D.vi"("Character 2D array"=w1233) -> ("U8 2D array"=w1232:u8[][])  [unwired: 10 in]
                  n569 = To Double Precision Float(number=w1232) -> (double precision float=w1231:dbl[][])
                  n570 = call-generic <vilib>:"NIMS_Get Scalar_w Error.vi"("A"=w1231) -> ("Error Enum"=w1219:T1, "Scalar"=w1234:dbl)  [unwired: 8 in, 1 out]
                  n571 = call-generic <vilib>:"NIMS_Complex To Real.vi"("A"=w1237) -> ("Error Enum"=w1221:T1, "Real(A)"=w1236:dbl[][])  [unwired: 8 in, 1 out]
                  n572 = To Long Integer(number=w1236) -> (32bit integer=w1235:i32[][])
                  n573 = call-generic <vilib>:"NIMS_Get Scalar_w Error.vi"("A"=w1235) -> ("Error Enum"=w1220:T1, "Scalar"=w1238:i32)  [unwired: 8 in, 1 out]
                  n574 = call-generic <vilib>:"NIMS_Complex To Real.vi"("A"=w1241) -> ("Error Enum"=w1223:T1, "Real(A)"=w1240:dbl[][])  [unwired: 8 in, 1 out]
                  n575 = To Long Integer(number=w1240) -> (32bit integer=w1239:i32[][])
                  n576 = call-generic <vilib>:"NIMS_Get Scalar_w Error.vi"("A"=w1239) -> ("Error Enum"=w1222:T1, "Scalar"=w1242:i32)  [unwired: 8 in, 1 out]
                  n577 = call <vilib>:"NIMS_DF_fir_nyquist(n,l,rf,non).vi"("flag"=w1230, "rolloff"=w1234, "l"=w1238, "n"=w1242) -> ("error"=w1215:i32, "b"=w1206:dbl[])  [unwired: 6 in]
                  n578 = Build Array(w1209, w1209, w1209, w1209, w1209, w1209, w1209, w1209, "fir_nyquist") -> (w1212:string[])
                  n579 = Build Array(w1223, w1222, w1221, w1220, w1219, w1218, w1217, w1216, w1215) -> (w1213:i32[])
                  n580 = call <vilib>:"NIMS_Create Error From Enums.vi"("Error Code"=bool[] [FALSE, FALSE, FALSE, FALSE, FALSE, FALSE, FALSE, FALSE, TRUE], "error in (no error)"=w1211, "Line no"=w1214, "Error Enums"=w1213, "Function names"=w1212) -> ("error out"=w1207:errorcluster)  [unwired: 6 in]
                }
                frame ";;_Char:Character;_Char:Character;" {
                  w1246 = "fir_nyquist"
                  n581 = call-generic <vilib>:"NIMS_Get Row Vector_w Error - Matrix.vi"("A"=w1262) -> ("Error Enum"=w1254:T1, "Row Vector"=w1261:T2[])  [unwired: 8 in, 1 out]
                  n582 = call <vilib>:"NIMS_CH_Character RV to String.vi"("Character array"=w1261) -> ("String"=w1263:string)  [unwired: 10 in]
                  n583 = call <vilib>:"NIMS_String to Enum.vi"("Input String"=w1263, "Enum choices"=string[] ["nonnegative"] ("Enum Options")) -> ("Error Enum"=w1253:T1, "Enum Index"=w1264:i32)  [unwired: 8 in]
                  n584 = call <vilib>:"NIMS_CH_Character 2D to U8 2D.vi"("Character 2D array"=w1267) -> ("U8 2D array"=w1266:u8[][])  [unwired: 10 in]
                  n585 = To Double Precision Float(number=w1266) -> (double precision float=w1265:dbl[][])
                  n586 = call-generic <vilib>:"NIMS_Get Scalar_w Error.vi"("A"=w1265) -> ("Error Enum"=w1255:T1, "Scalar"=w1268:dbl)  [unwired: 8 in, 1 out]
                  n587 = call-generic <vilib>:"NIMS_Complex To Real.vi"("A"=w1271) -> ("Error Enum"=w1257:T1, "Real(A)"=w1270:dbl[][])  [unwired: 8 in, 1 out]
                  n588 = To Long Integer(number=w1270) -> (32bit integer=w1269:i32[][])
                  n589 = call-generic <vilib>:"NIMS_Get Scalar_w Error.vi"("A"=w1269) -> ("Error Enum"=w1256:T1, "Scalar"=w1272:i32)  [unwired: 8 in, 1 out]
                  n590 = call-generic <vilib>:"NIMS_Complex To Real.vi"("A"=w1275) -> ("Error Enum"=w1259:T1, "Real(A)"=w1274:dbl[][])  [unwired: 8 in, 1 out]
                  n591 = To Long Integer(number=w1274) -> (32bit integer=w1273:i32[][])
                  n592 = call-generic <vilib>:"NIMS_Get Scalar_w Error.vi"("A"=w1273) -> ("Error Enum"=w1258:T1, "Scalar"=w1276:i32)  [unwired: 8 in, 1 out]
                  n593 = call <vilib>:"NIMS_DF_fir_nyquist(n,l,rf,non).vi"("flag"=w1264, "rolloff"=w1268, "l"=w1272, "n"=w1276) -> ("error"=w1252:i32, "b"=w1243:dbl[])  [unwired: 6 in]
                  n594 = Build Array(w1246, w1246, w1246, w1246, w1246, w1246, w1246, "fir_nyquist") -> (w1249:string[])
                  n595 = Build Array(w1259, w1258, w1257, w1256, w1255, w1254, w1253, w1252) -> (w1250:i32[])
                  n596 = call <vilib>:"NIMS_Create Error From Enums.vi"("Error Code"=bool[] [FALSE, FALSE, FALSE, FALSE, FALSE, FALSE, FALSE, TRUE], "error in (no error)"=w1248, "Line no"=w1251, "Error Enums"=w1250, "Function names"=w1249) -> ("error out"=w1244:errorcluster)  [unwired: 6 in]
                }
                frame ";_Char:Character;;;" {
                  w1280 = "fir_nyquist"
                  n597 = call-generic <vilib>:"NIMS_Complex To Real.vi"("A"=w1299) -> ("Error Enum"=w1289:T1, "Real(A)"=w1298:dbl[][])  [unwired: 8 in, 1 out]
                  n598 = To Unsigned Byte Integer(number=w1298) -> (unsigned 8bit integer=w1297:u8[][])
                  n599 = call-generic <vilib>:"NIMS_Get Row Vector_w Error - Matrix.vi"("A"=w1297) -> ("Error Enum"=w1288:T1, "Row Vector"=w1296:u8[])  [unwired: 8 in, 1 out]
                  n600 = Byte Array To String(unsigned byte array=w1296) -> (string=w1300:string)
                  n601 = call <vilib>:"NIMS_String to Enum.vi"("Input String"=w1300, "Enum choices"=string[] ["nonnegative"] ("Enum Options")) -> ("Error Enum"=w1287:T1, "Enum Index"=w1301:i32)  [unwired: 8 in]
                  n602 = call-generic <vilib>:"NIMS_Complex To Real.vi"("A"=w1303) -> ("Error Enum"=w1291:T1, "Real(A)"=w1302:dbl[][])  [unwired: 8 in, 1 out]
                  n603 = call-generic <vilib>:"NIMS_Get Scalar_w Error.vi"("A"=w1302) -> ("Error Enum"=w1290:T1, "Scalar"=w1304:dbl)  [unwired: 8 in, 1 out]
                  n604 = call <vilib>:"NIMS_CH_Character 2D to U8 2D.vi"("Character 2D array"=w1307) -> ("U8 2D array"=w1306:u8[][])  [unwired: 10 in]
                  n605 = To Long Integer(number=w1306) -> (32bit integer=w1305:i32[][])
                  n606 = call-generic <vilib>:"NIMS_Get Scalar_w Error.vi"("A"=w1305) -> ("Error Enum"=w1292:T1, "Scalar"=w1308:i32)  [unwired: 8 in, 1 out]
                  n607 = call-generic <vilib>:"NIMS_Complex To Real.vi"("A"=w1311) -> ("Error Enum"=w1294:T1, "Real(A)"=w1310:dbl[][])  [unwired: 8 in, 1 out]
                  n608 = To Long Integer(number=w1310) -> (32bit integer=w1309:i32[][])
                  n609 = call-generic <vilib>:"NIMS_Get Scalar_w Error.vi"("A"=w1309) -> ("Error Enum"=w1293:T1, "Scalar"=w1312:i32)  [unwired: 8 in, 1 out]
                  n610 = call <vilib>:"NIMS_DF_fir_nyquist(n,l,rf,non).vi"("flag"=w1301, "rolloff"=w1304, "l"=w1308, "n"=w1312) -> ("error"=w1286:i32, "b"=w1277:dbl[])  [unwired: 6 in]
                  n611 = Build Array(w1280, w1280, w1280, w1280, w1280, w1280, w1280, w1280, "fir_nyquist") -> (w1283:string[])
                  n612 = Build Array(w1294, w1293, w1292, w1291, w1290, w1289, w1288, w1287, w1286) -> (w1284:i32[])
                  n613 = call <vilib>:"NIMS_Create Error From Enums.vi"("Error Code"=bool[] [FALSE, FALSE, FALSE, FALSE, FALSE, FALSE, FALSE, FALSE, TRUE], "error in (no error)"=w1282, "Line no"=w1285, "Error Enums"=w1284, "Function names"=w1283) -> ("error out"=w1278:errorcluster)  [unwired: 6 in]
                }
                frame ";_Char:Character;;_Char:Character;" {
                  w1316 = "fir_nyquist"
                  n614 = call-generic <vilib>:"NIMS_Get Row Vector_w Error - Matrix.vi"("A"=w1332) -> ("Error Enum"=w1324:T1, "Row Vector"=w1331:T2[])  [unwired: 8 in, 1 out]
                  n615 = call <vilib>:"NIMS_CH_Character RV to String.vi"("Character array"=w1331) -> ("String"=w1333:string)  [unwired: 10 in]
                  n616 = call <vilib>:"NIMS_String to Enum.vi"("Input String"=w1333, "Enum choices"=string[] ["nonnegative"] ("Enum Options")) -> ("Error Enum"=w1323:T1, "Enum Index"=w1334:i32)  [unwired: 8 in]
                  n617 = call-generic <vilib>:"NIMS_Complex To Real.vi"("A"=w1336) -> ("Error Enum"=w1326:T1, "Real(A)"=w1335:dbl[][])  [unwired: 8 in, 1 out]
                  n618 = call-generic <vilib>:"NIMS_Get Scalar_w Error.vi"("A"=w1335) -> ("Error Enum"=w1325:T1, "Scalar"=w1337:dbl)  [unwired: 8 in, 1 out]
                  n619 = call <vilib>:"NIMS_CH_Character 2D to U8 2D.vi"("Character 2D array"=w1340) -> ("U8 2D array"=w1339:u8[][])  [unwired: 10 in]
                  n620 = To Long Integer(number=w1339) -> (32bit integer=w1338:i32[][])
                  n621 = call-generic <vilib>:"NIMS_Get Scalar_w Error.vi"("A"=w1338) -> ("Error Enum"=w1327:T1, "Scalar"=w1341:i32)  [unwired: 8 in, 1 out]
                  n622 = call-generic <vilib>:"NIMS_Complex To Real.vi"("A"=w1344) -> ("Error Enum"=w1329:T1, "Real(A)"=w1343:dbl[][])  [unwired: 8 in, 1 out]
                  n623 = To Long Integer(number=w1343) -> (32bit integer=w1342:i32[][])
                  n624 = call-generic <vilib>:"NIMS_Get Scalar_w Error.vi"("A"=w1342) -> ("Error Enum"=w1328:T1, "Scalar"=w1345:i32)  [unwired: 8 in, 1 out]
                  n625 = call <vilib>:"NIMS_DF_fir_nyquist(n,l,rf,non).vi"("flag"=w1334, "rolloff"=w1337, "l"=w1341, "n"=w1345) -> ("error"=w1322:i32, "b"=w1313:dbl[])  [unwired: 6 in]
                  n626 = Build Array(w1316, w1316, w1316, w1316, w1316, w1316, w1316, "fir_nyquist") -> (w1319:string[])
                  n627 = Build Array(w1329, w1328, w1327, w1326, w1325, w1324, w1323, w1322) -> (w1320:i32[])
                  n628 = call <vilib>:"NIMS_Create Error From Enums.vi"("Error Code"=bool[] [FALSE, FALSE, FALSE, FALSE, FALSE, FALSE, FALSE, TRUE], "error in (no error)"=w1318, "Line no"=w1321, "Error Enums"=w1320, "Function names"=w1319) -> ("error out"=w1314:errorcluster)  [unwired: 6 in]
                }
                frame ";_Char:Character;_Char:Character;;" {
                  w1349 = "fir_nyquist"
                  n629 = call-generic <vilib>:"NIMS_Complex To Real.vi"("A"=w1367) -> ("Error Enum"=w1358:T1, "Real(A)"=w1366:dbl[][])  [unwired: 8 in, 1 out]
                  n630 = To Unsigned Byte Integer(number=w1366) -> (unsigned 8bit integer=w1365:u8[][])
                  n631 = call-generic <vilib>:"NIMS_Get Row Vector_w Error - Matrix.vi"("A"=w1365) -> ("Error Enum"=w1357:T1, "Row Vector"=w1364:u8[])  [unwired: 8 in, 1 out]
                  n632 = Byte Array To String(unsigned byte array=w1364) -> (string=w1368:string)
                  n633 = call <vilib>:"NIMS_String to Enum.vi"("Input String"=w1368, "Enum choices"=string[] ["nonnegative"] ("Enum Options")) -> ("Error Enum"=w1356:T1, "Enum Index"=w1369:i32)  [unwired: 8 in]
                  n634 = call <vilib>:"NIMS_CH_Character 2D to U8 2D.vi"("Character 2D array"=w1372) -> ("U8 2D array"=w1371:u8[][])  [unwired: 10 in]
                  n635 = To Double Precision Float(number=w1371) -> (double precision float=w1370:dbl[][])
                  n636 = call-generic <vilib>:"NIMS_Get Scalar_w Error.vi"("A"=w1370) -> ("Error Enum"=w1359:T1, "Scalar"=w1373:dbl)  [unwired: 8 in, 1 out]
                  n637 = call <vilib>:"NIMS_CH_Character 2D to U8 2D.vi"("Character 2D array"=w1376) -> ("U8 2D array"=w1375:u8[][])  [unwired: 10 in]
                  n638 = To Long Integer(number=w1375) -> (32bit integer=w1374:i32[][])
                  n639 = call-generic <vilib>:"NIMS_Get Scalar_w Error.vi"("A"=w1374) -> ("Error Enum"=w1360:T1, "Scalar"=w1377:i32)  [unwired: 8 in, 1 out]
                  n640 = call-generic <vilib>:"NIMS_Complex To Real.vi"("A"=w1380) -> ("Error Enum"=w1362:T1, "Real(A)"=w1379:dbl[][])  [unwired: 8 in, 1 out]
                  n641 = To Long Integer(number=w1379) -> (32bit integer=w1378:i32[][])
                  n642 = call-generic <vilib>:"NIMS_Get Scalar_w Error.vi"("A"=w1378) -> ("Error Enum"=w1361:T1, "Scalar"=w1381:i32)  [unwired: 8 in, 1 out]
                  n643 = call <vilib>:"NIMS_DF_fir_nyquist(n,l,rf,non).vi"("flag"=w1369, "rolloff"=w1373, "l"=w1377, "n"=w1381) -> ("error"=w1355:i32, "b"=w1346:dbl[])  [unwired: 6 in]
                  n644 = Build Array(w1349, w1349, w1349, w1349, w1349, w1349, w1349, "fir_nyquist") -> (w1352:string[])
                  n645 = Build Array(w1362, w1361, w1360, w1359, w1358, w1357, w1356, w1355) -> (w1353:i32[])
                  n646 = call <vilib>:"NIMS_Create Error From Enums.vi"("Error Code"=bool[] [FALSE, FALSE, FALSE, FALSE, FALSE, FALSE, FALSE, TRUE], "error in (no error)"=w1351, "Line no"=w1354, "Error Enums"=w1353, "Function names"=w1352) -> ("error out"=w1347:errorcluster)  [unwired: 6 in]
                }
                frame ";_Char:Character;_Char:Character;_Char:Character;" {
                  w1385 = "fir_nyquist"
                  n647 = call-generic <vilib>:"NIMS_Get Row Vector_w Error - Matrix.vi"("A"=w1400) -> ("Error Enum"=w1393:T1, "Row Vector"=w1399:T2[])  [unwired: 8 in, 1 out]
                  n648 = call <vilib>:"NIMS_CH_Character RV to String.vi"("Character array"=w1399) -> ("String"=w1401:string)  [unwired: 10 in]
                  n649 = call <vilib>:"NIMS_String to Enum.vi"("Input String"=w1401, "Enum choices"=string[] ["nonnegative"] ("Enum Options")) -> ("Error Enum"=w1392:T1, "Enum Index"=w1402:i32)  [unwired: 8 in]
                  n650 = call <vilib>:"NIMS_CH_Character 2D to U8 2D.vi"("Character 2D array"=w1405) -> ("U8 2D array"=w1404:u8[][])  [unwired: 10 in]
                  n651 = To Double Precision Float(number=w1404) -> (double precision float=w1403:dbl[][])
                  n652 = call-generic <vilib>:"NIMS_Get Scalar_w Error.vi"("A"=w1403) -> ("Error Enum"=w1394:T1, "Scalar"=w1406:dbl)  [unwired: 8 in, 1 out]
                  n653 = call <vilib>:"NIMS_CH_Character 2D to U8 2D.vi"("Character 2D array"=w1409) -> ("U8 2D array"=w1408:u8[][])  [unwired: 10 in]
                  n654 = To Long Integer(number=w1408) -> (32bit integer=w1407:i32[][])
                  n655 = call-generic <vilib>:"NIMS_Get Scalar_w Error.vi"("A"=w1407) -> ("Error Enum"=w1395:T1, "Scalar"=w1410:i32)  [unwired: 8 in, 1 out]
                  n656 = call-generic <vilib>:"NIMS_Complex To Real.vi"("A"=w1413) -> ("Error Enum"=w1397:T1, "Real(A)"=w1412:dbl[][])  [unwired: 8 in, 1 out]
                  n657 = To Long Integer(number=w1412) -> (32bit integer=w1411:i32[][])
                  n658 = call-generic <vilib>:"NIMS_Get Scalar_w Error.vi"("A"=w1411) -> ("Error Enum"=w1396:T1, "Scalar"=w1414:i32)  [unwired: 8 in, 1 out]
                  n659 = call <vilib>:"NIMS_DF_fir_nyquist(n,l,rf,non).vi"("flag"=w1402, "rolloff"=w1406, "l"=w1410, "n"=w1414) -> ("error"=w1391:i32, "b"=w1382:dbl[])  [unwired: 6 in]
                  n660 = Build Array(w1385, w1385, w1385, w1385, w1385, w1385, "fir_nyquist") -> (w1388:string[])
                  n661 = Build Array(w1397, w1396, w1395, w1394, w1393, w1392, w1391) -> (w1389:i32[])
                  n662 = call <vilib>:"NIMS_Create Error From Enums.vi"("Error Code"=bool[] [FALSE, FALSE, FALSE, FALSE, FALSE, FALSE, TRUE], "error in (no error)"=w1387, "Line no"=w1390, "Error Enums"=w1389, "Function names"=w1388) -> ("error out"=w1383:errorcluster)  [unwired: 6 in]
                }
                frame "_Char:Character;;;;" {
                  w1418 = "fir_nyquist"
                  n663 = call-generic <vilib>:"NIMS_Complex To Real.vi"("A"=w1434) -> ("Error Enum"=w1426:T1, "Real(A)"=w1433:dbl[][])  [unwired: 8 in, 1 out]
                  n664 = call-generic <vilib>:"NIMS_Get Scalar_w Error.vi"("A"=w1433) -> ("Error Enum"=w1425:T1, "Scalar"=w1435:dbl)  [unwired: 8 in, 1 out]
                  n665 = call-generic <vilib>:"NIMS_Complex To Real.vi"("A"=w1437) -> ("Error Enum"=w1428:T1, "Real(A)"=w1436:dbl[][])  [unwired: 8 in, 1 out]
                  n666 = call-generic <vilib>:"NIMS_Get Scalar_w Error.vi"("A"=w1436) -> ("Error Enum"=w1427:T1, "Scalar"=w1438:dbl)  [unwired: 8 in, 1 out]
                  n667 = call-generic <vilib>:"NIMS_Complex To Real.vi"("A"=w1441) -> ("Error Enum"=w1430:T1, "Real(A)"=w1440:dbl[][])  [unwired: 8 in, 1 out]
                  n668 = To Long Integer(number=w1440) -> (32bit integer=w1439:i32[][])
                  n669 = call-generic <vilib>:"NIMS_Get Scalar_w Error.vi"("A"=w1439) -> ("Error Enum"=w1429:T1, "Scalar"=w1442:i32)  [unwired: 8 in, 1 out]
                  n670 = call-generic <vilib>:"NIMS_Get Row Vector_w Error - Matrix.vi"("A"=w1445) -> ("Error Enum"=w1432:T1, "Row Vector"=w1444:T2[])  [unwired: 8 in, 1 out]
                  n671 = call <vilib>:"NIMS_CH_Character RV to String.vi"("Character array"=w1444) -> ("String"=w1446:string)  [unwired: 10 in]
                  n672 = call <vilib>:"NIMS_String to Enum.vi"("Input String"=w1446, "Enum choices"=string[] ["minorder"] ("Enum Options")) -> ("Error Enum"=w1431:T1, "Enum Index"=w1447:i32)  [unwired: 8 in]
                  n673 = call <vilib>:"NIMS_DF_fir_nyquist(min,l,rf,ripple).vi"("ripple"=w1435, "rolloff"=w1438, "l"=w1442, "flag"=w1447) -> ("error"=w1424:i32, "b"=w1415:dbl[])  [unwired: 6 in]
                  n674 = Build Array(w1418, w1418, w1418, w1418, w1418, w1418, w1418, w1418, "fir_nyquist") -> (w1421:string[])
                  n675 = Build Array(w1432, w1431, w1430, w1429, w1428, w1427, w1426, w1425, w1424) -> (w1422:i32[])
                  n676 = call <vilib>:"NIMS_Create Error From Enums.vi"("Error Code"=bool[] [FALSE, FALSE, FALSE, FALSE, FALSE, FALSE, FALSE, FALSE, TRUE], "error in (no error)"=w1420, "Line no"=w1423, "Error Enums"=w1422, "Function names"=w1421) -> ("error out"=w1416:errorcluster)  [unwired: 6 in]
                }
                frame "_Char:Character;;;_Char:Character;" {
                  w1451 = "fir_nyquist"
                  n677 = call <vilib>:"NIMS_CH_Character 2D to U8 2D.vi"("Character 2D array"=w1467) -> ("U8 2D array"=w1466:u8[][])  [unwired: 10 in]
                  n678 = To Double Precision Float(number=w1466) -> (double precision float=w1465:dbl[][])
                  n679 = call-generic <vilib>:"NIMS_Get Scalar_w Error.vi"("A"=w1465) -> ("Error Enum"=w1458:T1, "Scalar"=w1468:dbl)  [unwired: 8 in, 1 out]
                  n680 = call-generic <vilib>:"NIMS_Complex To Real.vi"("A"=w1470) -> ("Error Enum"=w1460:T1, "Real(A)"=w1469:dbl[][])  [unwired: 8 in, 1 out]
                  n681 = call-generic <vilib>:"NIMS_Get Scalar_w Error.vi"("A"=w1469) -> ("Error Enum"=w1459:T1, "Scalar"=w1471:dbl)  [unwired: 8 in, 1 out]
                  n682 = call-generic <vilib>:"NIMS_Complex To Real.vi"("A"=w1474) -> ("Error Enum"=w1462:T1, "Real(A)"=w1473:dbl[][])  [unwired: 8 in, 1 out]
                  n683 = To Long Integer(number=w1473) -> (32bit integer=w1472:i32[][])
                  n684 = call-generic <vilib>:"NIMS_Get Scalar_w Error.vi"("A"=w1472) -> ("Error Enum"=w1461:T1, "Scalar"=w1475:i32)  [unwired: 8 in, 1 out]
                  n685 = call-generic <vilib>:"NIMS_Get Row Vector_w Error - Matrix.vi"("A"=w1478) -> ("Error Enum"=w1464:T1, "Row Vector"=w1477:T2[])  [unwired: 8 in, 1 out]
                  n686 = call <vilib>:"NIMS_CH_Character RV to String.vi"("Character array"=w1477) -> ("String"=w1479:string)  [unwired: 10 in]
                  n687 = call <vilib>:"NIMS_String to Enum.vi"("Input String"=w1479, "Enum choices"=string[] ["minorder"] ("Enum Options")) -> ("Error Enum"=w1463:T1, "Enum Index"=w1480:i32)  [unwired: 8 in]
                  n688 = call <vilib>:"NIMS_DF_fir_nyquist(min,l,rf,ripple).vi"("ripple"=w1468, "rolloff"=w1471, "l"=w1475, "flag"=w1480) -> ("error"=w1457:i32, "b"=w1448:dbl[])  [unwired: 6 in]
                  n689 = Build Array(w1451, w1451, w1451, w1451, w1451, w1451, w1451, "fir_nyquist") -> (w1454:string[])
                  n690 = Build Array(w1464, w1463, w1462, w1461, w1460, w1459, w1458, w1457) -> (w1455:i32[])
                  n691 = call <vilib>:"NIMS_Create Error From Enums.vi"("Error Code"=bool[] [FALSE, FALSE, FALSE, FALSE, FALSE, FALSE, FALSE, TRUE], "error in (no error)"=w1453, "Line no"=w1456, "Error Enums"=w1455, "Function names"=w1454) -> ("error out"=w1449:errorcluster)  [unwired: 6 in]
                }
                frame "_Char:Character;;_Char:Character;;" {
                  w1484 = "fir_nyquist"
                  n692 = call-generic <vilib>:"NIMS_Complex To Real.vi"("A"=w1499) -> ("Error Enum"=w1492:T1, "Real(A)"=w1498:dbl[][])  [unwired: 8 in, 1 out]
                  n693 = call-generic <vilib>:"NIMS_Get Scalar_w Error.vi"("A"=w1498) -> ("Error Enum"=w1491:T1, "Scalar"=w1500:dbl)  [unwired: 8 in, 1 out]
                  n694 = call <vilib>:"NIMS_CH_Character 2D to U8 2D.vi"("Character 2D array"=w1503) -> ("U8 2D array"=w1502:u8[][])  [unwired: 10 in]
                  n695 = To Double Precision Float(number=w1502) -> (double precision float=w1501:dbl[][])
                  n696 = call-generic <vilib>:"NIMS_Get Scalar_w Error.vi"("A"=w1501) -> ("Error Enum"=w1493:T1, "Scalar"=w1504:dbl)  [unwired: 8 in, 1 out]
                  n697 = call-generic <vilib>:"NIMS_Complex To Real.vi"("A"=w1507) -> ("Error Enum"=w1495:T1, "Real(A)"=w1506:dbl[][])  [unwired: 8 in, 1 out]
                  n698 = To Long Integer(number=w1506) -> (32bit integer=w1505:i32[][])
                  n699 = call-generic <vilib>:"NIMS_Get Scalar_w Error.vi"("A"=w1505) -> ("Error Enum"=w1494:T1, "Scalar"=w1508:i32)  [unwired: 8 in, 1 out]
                  n700 = call-generic <vilib>:"NIMS_Get Row Vector_w Error - Matrix.vi"("A"=w1511) -> ("Error Enum"=w1497:T1, "Row Vector"=w1510:T2[])  [unwired: 8 in, 1 out]
                  n701 = call <vilib>:"NIMS_CH_Character RV to String.vi"("Character array"=w1510) -> ("String"=w1512:string)  [unwired: 10 in]
                  n702 = call <vilib>:"NIMS_String to Enum.vi"("Input String"=w1512, "Enum choices"=string[] ["minorder"] ("Enum Options")) -> ("Error Enum"=w1496:T1, "Enum Index"=w1513:i32)  [unwired: 8 in]
                  n703 = call <vilib>:"NIMS_DF_fir_nyquist(min,l,rf,ripple).vi"("ripple"=w1500, "rolloff"=w1504, "l"=w1508, "flag"=w1513) -> ("error"=w1490:i32, "b"=w1481:dbl[])  [unwired: 6 in]
                  n704 = Build Array(w1484, w1484, w1484, w1484, w1484, w1484, w1484, "fir_nyquist") -> (w1487:string[])
                  n705 = Build Array(w1497, w1496, w1495, w1494, w1493, w1492, w1491, w1490) -> (w1488:i32[])
                  n706 = call <vilib>:"NIMS_Create Error From Enums.vi"("Error Code"=bool[] [FALSE, FALSE, FALSE, FALSE, FALSE, FALSE, FALSE, TRUE], "error in (no error)"=w1486, "Line no"=w1489, "Error Enums"=w1488, "Function names"=w1487) -> ("error out"=w1482:errorcluster)  [unwired: 6 in]
                }
                frame "_Char:Character;;_Char:Character;_Char:Character;" {
                  w1517 = "fir_nyquist"
                  n707 = call <vilib>:"NIMS_CH_Character 2D to U8 2D.vi"("Character 2D array"=w1532) -> ("U8 2D array"=w1531:u8[][])  [unwired: 10 in]
                  n708 = To Double Precision Float(number=w1531) -> (double precision float=w1530:dbl[][])
                  n709 = call-generic <vilib>:"NIMS_Get Scalar_w Error.vi"("A"=w1530) -> ("Error Enum"=w1524:T1, "Scalar"=w1533:dbl)  [unwired: 8 in, 1 out]
                  n710 = call <vilib>:"NIMS_CH_Character 2D to U8 2D.vi"("Character 2D array"=w1536) -> ("U8 2D array"=w1535:u8[][])  [unwired: 10 in]
                  n711 = To Double Precision Float(number=w1535) -> (double precision float=w1534:dbl[][])
                  n712 = call-generic <vilib>:"NIMS_Get Scalar_w Error.vi"("A"=w1534) -> ("Error Enum"=w1525:T1, "Scalar"=w1537:dbl)  [unwired: 8 in, 1 out]
                  n713 = call-generic <vilib>:"NIMS_Complex To Real.vi"("A"=w1540) -> ("Error Enum"=w1527:T1, "Real(A)"=w1539:dbl[][])  [unwired: 8 in, 1 out]
                  n714 = To Long Integer(number=w1539) -> (32bit integer=w1538:i32[][])
                  n715 = call-generic <vilib>:"NIMS_Get Scalar_w Error.vi"("A"=w1538) -> ("Error Enum"=w1526:T1, "Scalar"=w1541:i32)  [unwired: 8 in, 1 out]
                  n716 = call-generic <vilib>:"NIMS_Get Row Vector_w Error - Matrix.vi"("A"=w1544) -> ("Error Enum"=w1529:T1, "Row Vector"=w1543:T2[])  [unwired: 8 in, 1 out]
                  n717 = call <vilib>:"NIMS_CH_Character RV to String.vi"("Character array"=w1543) -> ("String"=w1545:string)  [unwired: 10 in]
                  n718 = call <vilib>:"NIMS_String to Enum.vi"("Input String"=w1545, "Enum choices"=string[] ["minorder"] ("Enum Options")) -> ("Error Enum"=w1528:T1, "Enum Index"=w1546:i32)  [unwired: 8 in]
                  n719 = call <vilib>:"NIMS_DF_fir_nyquist(min,l,rf,ripple).vi"("ripple"=w1533, "rolloff"=w1537, "l"=w1541, "flag"=w1546) -> ("error"=w1523:i32, "b"=w1514:dbl[])  [unwired: 6 in]
                  n720 = Build Array(w1517, w1517, w1517, w1517, w1517, w1517, "fir_nyquist") -> (w1520:string[])
                  n721 = Build Array(w1529, w1528, w1527, w1526, w1525, w1524, w1523) -> (w1521:i32[])
                  n722 = call <vilib>:"NIMS_Create Error From Enums.vi"("Error Code"=bool[] [FALSE, FALSE, FALSE, FALSE, FALSE, FALSE, TRUE], "error in (no error)"=w1519, "Line no"=w1522, "Error Enums"=w1521, "Function names"=w1520) -> ("error out"=w1515:errorcluster)  [unwired: 6 in]
                }
                frame "_Char:Character;_Char:Character;;;" {
                  w1550 = "fir_nyquist"
                  n723 = call-generic <vilib>:"NIMS_Complex To Real.vi"("A"=w1565) -> ("Error Enum"=w1558:T1, "Real(A)"=w1564:dbl[][])  [unwired: 8 in, 1 out]
                  n724 = call-generic <vilib>:"NIMS_Get Scalar_w Error.vi"("A"=w1564) -> ("Error Enum"=w1557:T1, "Scalar"=w1566:dbl)  [unwired: 8 in, 1 out]
                  n725 = call-generic <vilib>:"NIMS_Complex To Real.vi"("A"=w1568) -> ("Error Enum"=w1560:T1, "Real(A)"=w1567:dbl[][])  [unwired: 8 in, 1 out]
                  n726 = call-generic <vilib>:"NIMS_Get Scalar_w Error.vi"("A"=w1567) -> ("Error Enum"=w1559:T1, "Scalar"=w1569:dbl)  [unwired: 8 in, 1 out]
                  n727 = call <vilib>:"NIMS_CH_Character 2D to U8 2D.vi"("Character 2D array"=w1572) -> ("U8 2D array"=w1571:u8[][])  [unwired: 10 in]
                  n728 = To Long Integer(number=w1571) -> (32bit integer=w1570:i32[][])
                  n729 = call-generic <vilib>:"NIMS_Get Scalar_w Error.vi"("A"=w1570) -> ("Error Enum"=w1561:T1, "Scalar"=w1573:i32)  [unwired: 8 in, 1 out]
                  n730 = call-generic <vilib>:"NIMS_Get Row Vector_w Error - Matrix.vi"("A"=w1576) -> ("Error Enum"=w1563:T1, "Row Vector"=w1575:T2[])  [unwired: 8 in, 1 out]
                  n731 = call <vilib>:"NIMS_CH_Character RV to String.vi"("Character array"=w1575) -> ("String"=w1577:string)  [unwired: 10 in]
                  n732 = call <vilib>:"NIMS_String to Enum.vi"("Input String"=w1577, "Enum choices"=string[] ["minorder"] ("Enum Options")) -> ("Error Enum"=w1562:T1, "Enum Index"=w1578:i32)  [unwired: 8 in]
                  n733 = call <vilib>:"NIMS_DF_fir_nyquist(min,l,rf,ripple).vi"("ripple"=w1566, "rolloff"=w1569, "l"=w1573, "flag"=w1578) -> ("error"=w1556:i32, "b"=w1547:dbl[])  [unwired: 6 in]
                  n734 = Build Array(w1550, w1550, w1550, w1550, w1550, w1550, w1550, "fir_nyquist") -> (w1553:string[])
                  n735 = Build Array(w1563, w1562, w1561, w1560, w1559, w1558, w1557, w1556) -> (w1554:i32[])
                  n736 = call <vilib>:"NIMS_Create Error From Enums.vi"("Error Code"=bool[] [FALSE, FALSE, FALSE, FALSE, FALSE, FALSE, FALSE, TRUE], "error in (no error)"=w1552, "Line no"=w1555, "Error Enums"=w1554, "Function names"=w1553) -> ("error out"=w1548:errorcluster)  [unwired: 6 in]
                }
                frame "_Char:Character;_Char:Character;;_Char:Character;" {
                  w1582 = "fir_nyquist"
                  n737 = call <vilib>:"NIMS_CH_Character 2D to U8 2D.vi"("Character 2D array"=w1597) -> ("U8 2D array"=w1596:u8[][])  [unwired: 10 in]
                  n738 = To Double Precision Float(number=w1596) -> (double precision float=w1595:dbl[][])
                  n739 = call-generic <vilib>:"NIMS_Get Scalar_w Error.vi"("A"=w1595) -> ("Error Enum"=w1589:T1, "Scalar"=w1598:dbl)  [unwired: 8 in, 1 out]
                  n740 = call-generic <vilib>:"NIMS_Complex To Real.vi"("A"=w1600) -> ("Error Enum"=w1591:T1, "Real(A)"=w1599:dbl[][])  [unwired: 8 in, 1 out]
                  n741 = call-generic <vilib>:"NIMS_Get Scalar_w Error.vi"("A"=w1599) -> ("Error Enum"=w1590:T1, "Scalar"=w1601:dbl)  [unwired: 8 in, 1 out]
                  n742 = call <vilib>:"NIMS_CH_Character 2D to U8 2D.vi"("Character 2D array"=w1604) -> ("U8 2D array"=w1603:u8[][])  [unwired: 10 in]
                  n743 = To Long Integer(number=w1603) -> (32bit integer=w1602:i32[][])
                  n744 = call-generic <vilib>:"NIMS_Get Scalar_w Error.vi"("A"=w1602) -> ("Error Enum"=w1592:T1, "Scalar"=w1605:i32)  [unwired: 8 in, 1 out]
                  n745 = call-generic <vilib>:"NIMS_Get Row Vector_w Error - Matrix.vi"("A"=w1608) -> ("Error Enum"=w1594:T1, "Row Vector"=w1607:T2[])  [unwired: 8 in, 1 out]
                  n746 = call <vilib>:"NIMS_CH_Character RV to String.vi"("Character array"=w1607) -> ("String"=w1609:string)  [unwired: 10 in]
                  n747 = call <vilib>:"NIMS_String to Enum.vi"("Input String"=w1609, "Enum choices"=string[] ["minorder"] ("Enum Options")) -> ("Error Enum"=w1593:T1, "Enum Index"=w1610:i32)  [unwired: 8 in]
                  n748 = call <vilib>:"NIMS_DF_fir_nyquist(min,l,rf,ripple).vi"("ripple"=w1598, "rolloff"=w1601, "l"=w1605, "flag"=w1610) -> ("error"=w1588:i32, "b"=w1579:dbl[])  [unwired: 6 in]
                  n749 = Build Array(w1582, w1582, w1582, w1582, w1582, w1582, "fir_nyquist") -> (w1585:string[])
                  n750 = Build Array(w1594, w1593, w1592, w1591, w1590, w1589, w1588) -> (w1586:i32[])
                  n751 = call <vilib>:"NIMS_Create Error From Enums.vi"("Error Code"=bool[] [FALSE, FALSE, FALSE, FALSE, FALSE, FALSE, TRUE], "error in (no error)"=w1584, "Line no"=w1587, "Error Enums"=w1586, "Function names"=w1585) -> ("error out"=w1580:errorcluster)  [unwired: 6 in]
                }
                frame "_Char:Character;_Char:Character;_Char:Character;;" {
                  w1614 = "fir_nyquist"
                  n752 = call-generic <vilib>:"NIMS_Complex To Real.vi"("A"=w1628) -> ("Error Enum"=w1622:T1, "Real(A)"=w1627:dbl[][])  [unwired: 8 in, 1 out]
                  n753 = call-generic <vilib>:"NIMS_Get Scalar_w Error.vi"("A"=w1627) -> ("Error Enum"=w1621:T1, "Scalar"=w1629:dbl)  [unwired: 8 in, 1 out]
                  n754 = call <vilib>:"NIMS_CH_Character 2D to U8 2D.vi"("Character 2D array"=w1632) -> ("U8 2D array"=w1631:u8[][])  [unwired: 10 in]
                  n755 = To Double Precision Float(number=w1631) -> (double precision float=w1630:dbl[][])
                  n756 = call-generic <vilib>:"NIMS_Get Scalar_w Error.vi"("A"=w1630) -> ("Error Enum"=w1623:T1, "Scalar"=w1633:dbl)  [unwired: 8 in, 1 out]
                  n757 = call <vilib>:"NIMS_CH_Character 2D to U8 2D.vi"("Character 2D array"=w1636) -> ("U8 2D array"=w1635:u8[][])  [unwired: 10 in]
                  n758 = To Long Integer(number=w1635) -> (32bit integer=w1634:i32[][])
                  n759 = call-generic <vilib>:"NIMS_Get Scalar_w Error.vi"("A"=w1634) -> ("Error Enum"=w1624:T1, "Scalar"=w1637:i32)  [unwired: 8 in, 1 out]
                  n760 = call-generic <vilib>:"NIMS_Get Row Vector_w Error - Matrix.vi"("A"=w1640) -> ("Error Enum"=w1626:T1, "Row Vector"=w1639:T2[])  [unwired: 8 in, 1 out]
                  n761 = call <vilib>:"NIMS_CH_Character RV to String.vi"("Character array"=w1639) -> ("String"=w1641:string)  [unwired: 10 in]
                  n762 = call <vilib>:"NIMS_String to Enum.vi"("Input String"=w1641, "Enum choices"=string[] ["minorder"] ("Enum Options")) -> ("Error Enum"=w1625:T1, "Enum Index"=w1642:i32)  [unwired: 8 in]
                  n763 = call <vilib>:"NIMS_DF_fir_nyquist(min,l,rf,ripple).vi"("ripple"=w1629, "rolloff"=w1633, "l"=w1637, "flag"=w1642) -> ("error"=w1620:i32, "b"=w1611:dbl[])  [unwired: 6 in]
                  n764 = Build Array(w1614, w1614, w1614, w1614, w1614, w1614, "fir_nyquist") -> (w1617:string[])
                  n765 = Build Array(w1626, w1625, w1624, w1623, w1622, w1621, w1620) -> (w1618:i32[])
                  n766 = call <vilib>:"NIMS_Create Error From Enums.vi"("Error Code"=bool[] [FALSE, FALSE, FALSE, FALSE, FALSE, FALSE, TRUE], "error in (no error)"=w1616, "Line no"=w1619, "Error Enums"=w1618, "Function names"=w1617) -> ("error out"=w1612:errorcluster)  [unwired: 6 in]
                }
                frame "_Char:Character;_Char:Character;_Char:Character;_Char:Character;" {
                  w1646 = "fir_nyquist"
                  n767 = call <vilib>:"NIMS_CH_Character 2D to U8 2D.vi"("Character 2D array"=w1660) -> ("U8 2D array"=w1659:u8[][])  [unwired: 10 in]
                  n768 = To Double Precision Float(number=w1659) -> (double precision float=w1658:dbl[][])
                  n769 = call-generic <vilib>:"NIMS_Get Scalar_w Error.vi"("A"=w1658) -> ("Error Enum"=w1653:T1, "Scalar"=w1661:dbl)  [unwired: 8 in, 1 out]
                  n770 = call <vilib>:"NIMS_CH_Character 2D to U8 2D.vi"("Character 2D array"=w1664) -> ("U8 2D array"=w1663:u8[][])  [unwired: 10 in]
                  n771 = To Double Precision Float(number=w1663) -> (double precision float=w1662:dbl[][])
                  n772 = call-generic <vilib>:"NIMS_Get Scalar_w Error.vi"("A"=w1662) -> ("Error Enum"=w1654:T1, "Scalar"=w1665:dbl)  [unwired: 8 in, 1 out]
                  n773 = call <vilib>:"NIMS_CH_Character 2D to U8 2D.vi"("Character 2D array"=w1668) -> ("U8 2D array"=w1667:u8[][])  [unwired: 10 in]
                  n774 = To Long Integer(number=w1667) -> (32bit integer=w1666:i32[][])
                  n775 = call-generic <vilib>:"NIMS_Get Scalar_w Error.vi"("A"=w1666) -> ("Error Enum"=w1655:T1, "Scalar"=w1669:i32)  [unwired: 8 in, 1 out]
                  n776 = call-generic <vilib>:"NIMS_Get Row Vector_w Error - Matrix.vi"("A"=w1672) -> ("Error Enum"=w1657:T1, "Row Vector"=w1671:T2[])  [unwired: 8 in, 1 out]
                  n777 = call <vilib>:"NIMS_CH_Character RV to String.vi"("Character array"=w1671) -> ("String"=w1673:string)  [unwired: 10 in]
                  n778 = call <vilib>:"NIMS_String to Enum.vi"("Input String"=w1673, "Enum choices"=string[] ["minorder"] ("Enum Options")) -> ("Error Enum"=w1656:T1, "Enum Index"=w1674:i32)  [unwired: 8 in]
                  n779 = call <vilib>:"NIMS_DF_fir_nyquist(min,l,rf,ripple).vi"("ripple"=w1661, "rolloff"=w1665, "l"=w1669, "flag"=w1674) -> ("error"=w1652:i32, "b"=w1643:dbl[])  [unwired: 6 in]
                  n780 = Build Array(w1646, w1646, w1646, w1646, w1646, "fir_nyquist") -> (w1649:string[])
                  n781 = Build Array(w1657, w1656, w1655, w1654, w1653, w1652) -> (w1650:i32[])
                  n782 = call <vilib>:"NIMS_Create Error From Enums.vi"("Error Code"=bool[] [FALSE, FALSE, FALSE, FALSE, FALSE, TRUE], "error in (no error)"=w1648, "Line no"=w1651, "Error Enums"=w1650, "Function names"=w1649) -> ("error out"=w1644:errorcluster)  [unwired: 6 in]
                }
              }
              n783 = Build Array(w1104) -> (w1103:dbl[][])
              n784 = To Double Precision Complex(1:w1103) -> (0:w1102:cdb[][])
              n785 = call-generic <vilib>:"NIMS_RunTimeType_From StrictType (excl LVString).vi"("Plug-In Name"="", "Data In"=w1102) -> ("Data Out"=w1100:variant)  [unwired: 2 in]
              n786 = Build Array(w1100) -> (w1099:variant[])
            }
          }
        }
      }
    }
    frame Error {
    }
  }
  "error out" <- w3
  "[funct(A)]" <- w4
